vi "CFM_DAQ.vi"() -> ()   [LabVIEW 2012]
panel:
  in  "stop":bool
  out "reinicio":bool
  out "M54":bool
  out "M53":bool
  out "M52":bool
  out "M51":bool
  in  "ACTUADOR RECHAZO":bool
  out "M50":bool
  out "M49":bool
  out "M48":bool
  out "M47":bool
  out "M46":bool
  out "M45":bool
  out "M44":bool
  out "TAPA NOPESO":bool
  out "M43":bool
  out "M42":bool
  out "M41":bool
  out "M40":bool
  out "M39":bool
  out "M38":bool
  out "M37":bool
  out "M36":bool
  out "M35":bool
  out "M34":bool
  out "TARRO NOPESO":bool
  out "DEPOSITO NOPESO":bool
  out "TAPA NOCOLOR":bool
  out "TARRO NOCOLOR":bool
  out "DEPOSITO NOCOLOR":bool
  out "CILINDRO RECHAZO1":bool
  out "VASTAGO RECHAZO":bool
  out "PINZA CERRADA":bool
  in  "PINZA ABIERTA":bool
  out "CILINDRO RECHAZO":bool
  out "ESTRUCTURA RECHAZO":bool
  out "M33":bool
  out "M32":bool
  out "M31":bool
  out "M30":bool
  out "M29":bool
  out "M28":bool
  out "M27":bool
  out "M26":bool
  out "TAPA AZUL":bool
  out "M25":bool
  out "M24":bool
  out "TAPA TARRO ROJO":bool
  in  "CILINDRO MODULO6":bool
  in  "VASTAGO MODULO6":bool
  in  "MODULO6":bool
  out "M23":bool
  out "M22":bool
  out "M21":bool
  out "ANALIZANDO\nCC":bool
  out "M20":bool
  out "balanza2":bool
  out "M19":bool
  out "M18":bool
  out "M17":bool
  out "M16":bool
  out "M15":bool
  out "M14":bool
  out "M13":bool
  out "M12":bool
  out "M11":bool
  out "M10":bool
  out "M9":bool
  out "M8":bool
  out "M7":bool
  out "M6":bool
  out "M5":bool
  out "M4":bool
  out "M3":bool
  out "M2":bool
  out "M1":bool
  out "tapa neutrop":bool
  out "cilindro3 tapado":bool
  out "vastago3 tapado":bool
  out "vastago4 tapado":bool
  out "cilindro2 tapado":bool
  in  "vastago2 tapado":bool
  out "cilindro1 tapado":bool
  in  "vastago1 tapado":bool
  out "estructura tapado":bool
  out "tarro llenop":bool
  out "tarro vaciop1":bool
  out "cilindros tolva":bool
  out "perta tolva1":bool
  out "puerta tolva2":bool
  out "dep inferior":bool
  out "dep superior":bool
  out "tolva vacia":bool
  out "cuadroblanco":bool
  out "vastagoaux1":bool
  out "tarro vaciop":bool
  out "estructura1":bool
  out "CILINDRO NUEVO":bool
  out "TAPA NEUTRO":bool
  out "BALANZA1":bool
  in  "BASTAGO TAPAS":bool
  out "PUERTA TOLVA":bool
  out "CAJA LLENA":bool
  out "TARRO VACIO":bool
  in  "BPESO NO":bool
  in  "BPESO SI":bool
  in  "BNO COLOR":bool
  in  "BROJO":bool
  in  "BAZUL":bool
  in  "REINICIAR\nCONTEO":bool
  out "FINALIZADOS\nRECHAZADOS":dbl
  out "FINALIZADOS\nROJOS":dbl
  out "FINALIZADOS\nAZULES":dbl
  out "AZUL":bool
  out "ROJO":bool
  out "NO \nCOLOR":bool
  out "PESO\nNO":bool
  out "PESO\nSI":bool
  in  "RESET":bool
  in  "INICIO":bool
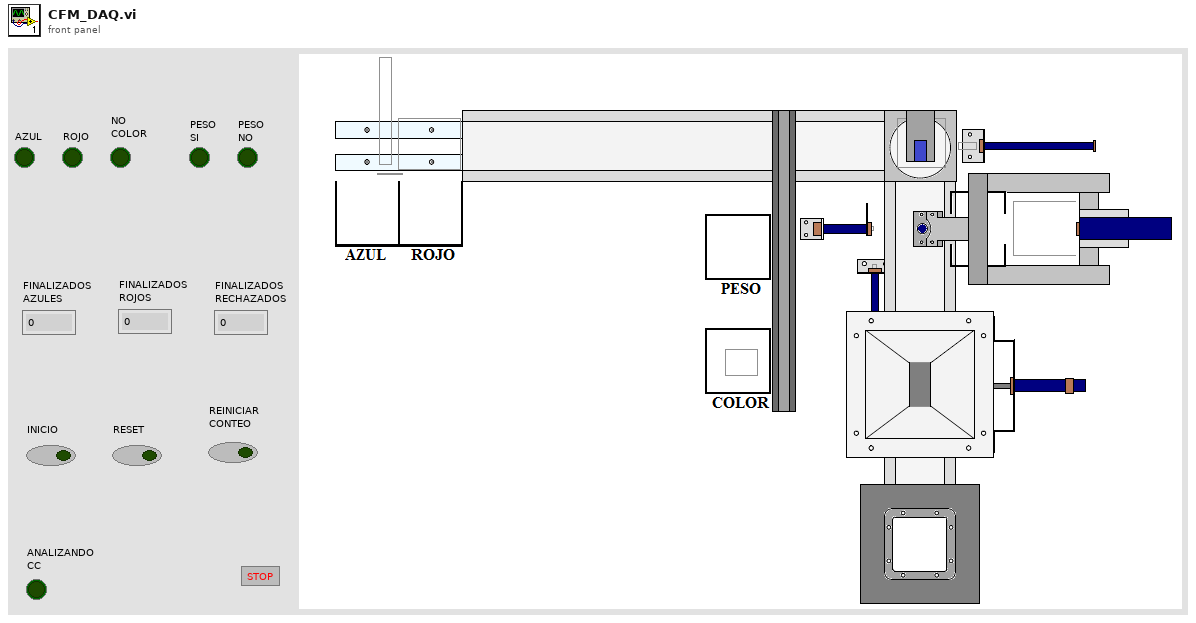
[diagram p1: front panel]
diagram:
  n1 = while {
    stop <- "stop" stop-if-true
    n2 = property on="M53" class="Bool (strict)"("Visible"=FALSE) -> ()  [unwired: 2 in, 2 out]
    n3 = property on="M54" class="Bool (strict)"("Visible"=FALSE) -> ()  [unwired: 2 in, 2 out]
    n4 = property on="M52" class="Bool (strict)"("Visible"=FALSE) -> ()  [unwired: 2 in, 2 out]
    n5 = property on="M48" class="Bool (strict)"("Visible"=FALSE) -> ()  [unwired: 2 in, 2 out]
    n6 = property on="M43" class="Bool (strict)"("Visible"=FALSE) -> ()  [unwired: 2 in, 2 out]
    n7 = property on="M47" class="Bool (strict)"("Visible"=FALSE) -> ()  [unwired: 2 in, 2 out]
    n8 = property on="M42" class="Bool (strict)"("Visible"=FALSE) -> ()  [unwired: 2 in, 2 out]
    n9 = property on="M41" class="Bool (strict)"("Visible"=FALSE) -> ()  [unwired: 2 in, 2 out]
    n10 = property on="M49" class="Bool (strict)"("Visible"=FALSE) -> ()  [unwired: 2 in, 2 out]
    n11 = property on="M40" class="Bool (strict)"("Visible"=FALSE) -> ()  [unwired: 2 in, 2 out]
    n12 = property on="M45" class="Bool (strict)"("Visible"=FALSE) -> ()  [unwired: 2 in, 2 out]
    n13 = property on="M46" class="Bool (strict)"("Visible"=FALSE) -> ()  [unwired: 2 in, 2 out]
    n14 = property on="reinicio" class="Bool (strict)"("Visible"=FALSE) -> ()  [unwired: 2 in, 2 out]
    n15 = property on="M24" class="Bool (strict)"("Visible"=FALSE) -> ()  [unwired: 2 in, 2 out]
    n16 = property on="M39" class="Bool (strict)"("Visible"=FALSE) -> ()  [unwired: 2 in, 2 out]
    n17 = property on="M44" class="Bool (strict)"("Visible"=FALSE) -> ()  [unwired: 2 in, 2 out]
    n18 = property on="M50" class="Bool (strict)"("Visible"=FALSE) -> ()  [unwired: 2 in, 2 out]
    n19 = property on="M25" class="Bool (strict)"("Visible"=FALSE) -> ()  [unwired: 2 in, 2 out]
    n20 = property on="M37" class="Bool (strict)"("Visible"=FALSE) -> ()  [unwired: 2 in, 2 out]
    n21 = property on="M38" class="Bool (strict)"("Visible"=FALSE) -> ()  [unwired: 2 in, 2 out]
    n22 = property on="M23" class="Bool (strict)"("Visible"=FALSE) -> ()  [unwired: 2 in, 2 out]
    n23 = property on="M22" class="Bool (strict)"("Visible"=FALSE) -> ()  [unwired: 2 in, 2 out]
    n24 = property on="M51" class="Bool (strict)"("Visible"=FALSE) -> ()  [unwired: 2 in, 2 out]
    n25 = property on="M36" class="Bool (strict)"("Visible"=FALSE) -> ()  [unwired: 2 in, 2 out]
    n26 = property on="M21" class="Bool (strict)"("Visible"=FALSE) -> ()  [unwired: 2 in, 2 out]
    n27 = property on="M27" class="Bool (strict)"("Visible"=FALSE) -> ()  [unwired: 2 in, 2 out]
    n28 = property on="M33" class="Bool (strict)"("Visible"=FALSE) -> ()  [unwired: 2 in, 2 out]
    n29 = property on="M2" class="Bool (strict)"("Visible"=FALSE) -> ()  [unwired: 2 in, 2 out]
    n30 = property on="M26" class="Bool (strict)"("Visible"=FALSE) -> ()  [unwired: 2 in, 2 out]
    n31 = property on="M35" class="Bool (strict)"("Visible"=FALSE) -> ()  [unwired: 2 in, 2 out]
    n32 = property on="M1" class="Bool (strict)"("Visible"=FALSE) -> ()  [unwired: 2 in, 2 out]
    n33 = property on="M32" class="Bool (strict)"("Visible"=FALSE) -> ()  [unwired: 2 in, 2 out]
    n34 = property on="M34" class="Bool (strict)"("Visible"=FALSE) -> ()  [unwired: 2 in, 2 out]
    n35 = property on="M13" class="Bool (strict)"("Visible"=FALSE) -> ()  [unwired: 2 in, 2 out]
    n36 = property on="M20" class="Bool (strict)"("Visible"=FALSE) -> ()  [unwired: 2 in, 2 out]
    n37 = property on="M29" class="Bool (strict)"("Visible"=FALSE) -> ()  [unwired: 2 in, 2 out]
    n38 = property on="M15" class="Bool (strict)"("Visible"=FALSE) -> ()  [unwired: 2 in, 2 out]
    n39 = property on="M28" class="Bool (strict)"("Visible"=FALSE) -> ()  [unwired: 2 in, 2 out]
    n40 = property on="M5" class="Bool (strict)"("Visible"=FALSE) -> ()  [unwired: 2 in, 2 out]
    n41 = property on="M3" class="Bool (strict)"("Visible"=FALSE) -> ()  [unwired: 2 in, 2 out]
    n42 = property on="M18" class="Bool (strict)"("Visible"=FALSE) -> ()  [unwired: 2 in, 2 out]
    n43 = property on="M19" class="Bool (strict)"("Visible"=FALSE) -> ()  [unwired: 2 in, 2 out]
    n44 = property on="M8" class="Bool (strict)"("Visible"=FALSE) -> ()  [unwired: 2 in, 2 out]
    n45 = property on="M7" class="Bool (strict)"("Visible"=FALSE) -> ()  [unwired: 2 in, 2 out]
    n46 = property on="M30" class="Bool (strict)"("Visible"=FALSE) -> ()  [unwired: 2 in, 2 out]
    n47 = property on="M6" class="Bool (strict)"("Visible"=FALSE) -> ()  [unwired: 2 in, 2 out]
    n48 = property on="M9" class="Bool (strict)"("Visible"=FALSE) -> ()  [unwired: 2 in, 2 out]
    n49 = property on="M17" class="Bool (strict)"("Visible"=FALSE) -> ()  [unwired: 2 in, 2 out]
    n50 = property on="M4" class="Bool (strict)"("Visible"=FALSE) -> ()  [unwired: 2 in, 2 out]
    n51 = property on="M10" class="Bool (strict)"("Visible"=FALSE) -> ()  [unwired: 2 in, 2 out]
    n52 = property on="M11" class="Bool (strict)"("Visible"=FALSE) -> ()  [unwired: 2 in, 2 out]
    n53 = property on="M14" class="Bool (strict)"("Visible"=FALSE) -> ()  [unwired: 2 in, 2 out]
    n54 = property on="M16" class="Bool (strict)"("Visible"=FALSE) -> ()  [unwired: 2 in, 2 out]
    n55 = property on="M12" class="Bool (strict)"("Visible"=FALSE) -> ()  [unwired: 2 in, 2 out]
    n56 = property on="M31" class="Bool (strict)"("Visible"=FALSE) -> ()  [unwired: 2 in, 2 out]
    n57 = property on="ACTUADOR RECHAZO" class="Bool (strict)"() -> ("Top"=w101:i32)  [unwired: 2 in, 2 out]
    n58 = property on="ACTUADOR RECHAZO" class="Bool (strict)"() -> ("Top"=w86:i32)  [unwired: 2 in, 2 out]
    n59 = local read "BNO COLOR"() -> (w140:bool)
    n60 = property on="ACTUADOR RECHAZO" class="Bool (strict)"() -> ("Top"=w116:i32)  [unwired: 2 in, 2 out]
    n61 = property on="ACTUADOR RECHAZO" class="Bool (strict)"() -> ("Top"=w173:i32)  [unwired: 2 in, 2 out]
    n62 = property on="ACTUADOR RECHAZO" class="Bool (strict)"() -> ("Top"=w158:i32)  [unwired: 2 in, 2 out]
    n63 = property on="VASTAGO MODULO6" class="Bool (strict)"() -> ("Top"=w251:i32)  [unwired: 2 in, 2 out]
    n64 = property on="VASTAGO MODULO6" class="Bool (strict)"() -> ("Top"=w214:i32)  [unwired: 2 in, 2 out]
    n65 = property on="VASTAGO MODULO6" class="Bool (strict)"() -> ("Top"=w209:i32)  [unwired: 2 in, 2 out]
    n66 = property on="VASTAGO MODULO6" class="Bool (strict)"() -> ("Top"=w256:i32)  [unwired: 2 in, 2 out]
    n67 = local read "BPESO NO"() -> (w141:bool)
    n68 = local read "BPESO NO"() -> (w187:bool)
    n69 = property on="TAPA TARRO ROJO" class="Bool (strict)"() -> ("Left"=w261:i32)  [unwired: 2 in, 2 out]
    n70 = property on="PINZA CERRADA" class="Bool (strict)"() -> ("Top"=w96:i32)  [unwired: 2 in, 2 out]
    n71 = property on="PINZA CERRADA" class="Bool (strict)"() -> ("Top"=w148:i32)  [unwired: 2 in, 2 out]
    n72 = property on="PINZA CERRADA" class="Bool (strict)"() -> ("Top"=w106:i32)  [unwired: 2 in, 2 out]
    n73 = property on="PINZA CERRADA" class="Bool (strict)"() -> ("Top"=w91:i32)  [unwired: 2 in, 2 out]
    n74 = property on="vastago4 tapado" class="Bool (strict)"() -> ("Top"=w319:i32)  [unwired: 2 in, 2 out]
    n75 = property on="PINZA CERRADA" class="Bool (strict)"() -> ("Top"=w168:i32)  [unwired: 2 in, 2 out]
    n76 = property on="PINZA CERRADA" class="Bool (strict)"() -> ("Top"=w163:i32)  [unwired: 2 in, 2 out]
    n77 = property on="vastago4 tapado" class="Bool (strict)"() -> ("Top"=w314:i32)  [unwired: 2 in, 2 out]
    n78 = property on="TAPA NOCOLOR" class="Bool (strict)"() -> ("Left"=w178:i32)  [unwired: 2 in, 2 out]
    n79 = property on="PINZA CERRADA" class="Bool (strict)"() -> ("Top"=w111:i32)  [unwired: 2 in, 2 out]
    n80 = property on="BASTAGO TAPAS" class="Bool (strict)"() -> ("Left"=w324:i32)  [unwired: 2 in, 2 out]
    n81 = local read "BNO COLOR"() -> (w188:bool)
    n82 = property on="CILINDRO NUEVO" class="Bool (strict)"() -> ("Left"=w309:i32)  [unwired: 2 in, 2 out]
    n83 = property on="vastago3 tapado" class="Bool (strict)"() -> ("Top"=w299:i32)  [unwired: 2 in, 2 out]
    n84 = property on="PINZA CERRADA" class="Bool (strict)"() -> ("Top"=w153:i32)  [unwired: 2 in, 2 out]
    n85 = property on="TAPA NOPESO" class="Bool (strict)"() -> ("Left"=w121:i32)  [unwired: 2 in, 2 out]
    n86 = property on="TAPA NEUTRO" class="Bool (strict)"() -> ("Top"=w294:i32)  [unwired: 2 in, 2 out]
    n87 = property on="balanza2" class="Bool (strict)"() -> ("Left"=w128:i32)  [unwired: 2 in, 2 out]
    n88 = property on="TAPA NEUTRO" class="Bool (strict)"() -> ("Top"=w284:i32)  [unwired: 2 in, 2 out]
    n89 = property on="tapa neutrop" class="Bool (strict)"() -> ("Top"=w304:i32)  [unwired: 2 in, 2 out]
    n90 = property on="PUERTA TOLVA" class="Bool (strict)"() -> ("Left"=w349:i32)  [unwired: 2 in, 2 out]
    n91 = property on="PUERTA TOLVA" class="Bool (strict)"() -> ("Left"=w344:i32)  [unwired: 2 in, 2 out]
    n92 = call "DAQ Assistant"() -> ("data"=w76:bool[])  [unwired: 17 in, 2 out]
    n93 = property on="TARRO VACIO" class="Bool (strict)"() -> ("Top"=w354:i32)  [unwired: 2 in, 2 out]
    n94 = property on="vastagoaux1" class="Bool (strict)"() -> ("Top"=w364:i32)  [unwired: 2 in, 2 out]
    n95 = local read "BPESO SI"() -> (w243:bool)
    n96 = local read "BPESO NO"() -> (w143:bool)
    n97 = property on="balanza2" class="Bool (strict)"() -> ("Left"=w138:i32)  [unwired: 2 in, 2 out]
    n98 = local read "BPESO SI"() -> (w249:bool)
    n99 = property on="vastagoaux1" class="Bool (strict)"() -> ("Top"=w369:i32)  [unwired: 2 in, 2 out]
    n100 = property on="vastagoaux1" class="Bool (strict)"() -> ("Top"=w359:i32)  [unwired: 2 in, 2 out]
    n101 = property on="puerta tolva2" class="Bool (strict)"() -> ("Left"=w339:i32)  [unwired: 2 in, 2 out]
    n102 = property on="puerta tolva2" class="Bool (strict)"() -> ("Left"=w334:i32)  [unwired: 2 in, 2 out]
    n103 = property on="TAPA AZUL" class="Bool (strict)"() -> ("Left"=w224:i32)  [unwired: 2 in, 2 out]
    n104 = property on="CAJA LLENA" class="Bool (strict)"() -> ("Top"=w329:i32)  [unwired: 2 in, 2 out]
    n105 = property on="BALANZA1" class="Bool (strict)"() -> ("Top"=w289:i32)  [unwired: 2 in, 2 out]
    n106 = property on="MODULO6" class="Bool (strict)"() -> ("Left"=w219:i32)  [unwired: 2 in, 2 out]
    n107 = property on="MODULO6" class="Bool (strict)"() -> ("Left"=w204:i32)  [unwired: 2 in, 2 out]
    n108 = local read "BAZUL"() -> (w244:bool)
    n109 = property on="balanza2" class="Bool (strict)"() -> ("Left"=w133:i32)  [unwired: 2 in, 2 out]
    n110 = local read "BROJO"() -> (w248:bool)
    n111 = property on="balanza2" class="Bool (strict)"() -> ("Left"=w239:i32)  [unwired: 2 in, 2 out]
    n112 = property on="balanza2" class="Bool (strict)"() -> ("Left"=w278:i32)  [unwired: 2 in, 2 out]
    n113 = property on="balanza2" class="Bool (strict)"() -> ("Left"=w183:i32)  [unwired: 2 in, 2 out]
    n114 = property on="balanza2" class="Bool (strict)"() -> ("Left"=w229:i32)  [unwired: 2 in, 2 out]
    n115 = property on="balanza2" class="Bool (strict)"() -> ("Left"=w195:i32)  [unwired: 2 in, 2 out]
    n116 = property on="balanza2" class="Bool (strict)"() -> ("Left"=w266:i32)  [unwired: 2 in, 2 out]
    n117 = property on="balanza2" class="Bool (strict)"() -> ("Left"=w234:i32)  [unwired: 2 in, 2 out]
    n118 = property on="balanza2" class="Bool (strict)"() -> ("Left"=w190:i32)  [unwired: 2 in, 2 out]
    n119 = property on="balanza2" class="Bool (strict)"() -> ("Left"=w271:i32)  [unwired: 2 in, 2 out]
    n120 = local read "reinicio"() -> (w82:bool)
    n121 = local read "INICIO"() -> (w83:bool)
    n122 = Not(x=w187) -> (.not. x?=w199:bool)
    n123 = local read "M46"() -> (w125:bool)
    n124 = And(x=w141, y=w140) -> (x .and. y?=w142:bool)
    n125 = Less?(x=w138, y=965) -> (x < y?=w139:bool)
    n126 = local read "M52"() -> (w98:bool)
    n127 = local read "M47"() -> (w123:bool)
    n128 = local read "M45"() -> (w130:bool)
    n129 = local read "M43"() -> (w150:bool)
    n130 = local read "M50"() -> (w108:bool)
    n131 = local read "M44"() -> (w135:bool)
    n132 = local read "M51"() -> (w103:bool)
    n133 = local read "M54"() -> (w88:bool)
    n134 = local read "M19"() -> (w281:bool)
    n135 = local read "M25"() -> (w253:bool)
    n136 = local read "M26"() -> (w241:bool)
    n137 = local read "M36"() -> (w185:bool)
    n138 = local read "M37"() -> (w180:bool)
    n139 = Greater?(x=w128, y=977) -> (0:w129:bool)
    n140 = local read "M53"() -> (w93:bool)
    n141 = local read "M28"() -> (w231:bool)
    n142 = local read "M48"() -> (w118:bool)
    n143 = local read "M10"() -> (w326:bool)
    n144 = local read "M14"() -> (w306:bool)
    n145 = local read "M16"() -> (w296:bool)
    n146 = local read "M20"() -> (w276:bool)
    n147 = local read "M30"() -> (w221:bool)
    n148 = local read "M31"() -> (w216:bool)
    n149 = local read "M33"() -> (w206:bool)
    n150 = local read "M39"() -> (w170:bool)
    n151 = local read "M40"() -> (w165:bool)
    n152 = local read "M23"() -> (w263:bool)
    n153 = local read "M29"() -> (w226:bool)
    n154 = local read "M34"() -> (w197:bool)
    n155 = local read "M41"() -> (w160:bool)
    n156 = local read "M12"() -> (w316:bool)
    n157 = local read "M19"() -> (w246:bool)
    n158 = local read "M32"() -> (w211:bool)
    n159 = local read "M19"() -> (w201:bool)
    n160 = local read "M38"() -> (w175:bool)
    n161 = local read "M49"() -> (w113:bool)
    n162 = local read "M11"() -> (w321:bool)
    n163 = local read "M17"() -> (w291:bool)
    n164 = local read "M18"() -> (w286:bool)
    n165 = local read "M22"() -> (w268:bool)
    n166 = local read "M24"() -> (w258:bool)
    n167 = local read "M27"() -> (w236:bool)
    n168 = local read "M35"() -> (w192:bool)
    n169 = local read "M42"() -> (w155:bool)
    n170 = local read "M19"() -> (w145:bool)
    n171 = local read "M2"() -> (w366:bool)
    n172 = local read "M15"() -> (w301:bool)
    n173 = local read "M1"() -> (w371:bool)
    n174 = local read "M21"() -> (w273:bool)
    n175 = local read "M4"() -> (w356:bool)
    n176 = local read "M13"() -> (w311:bool)
    n177 = local read "M6"() -> (w346:bool)
    n178 = local read "M8"() -> (w336:bool)
    n179 = local read "M3"() -> (w361:bool)
    n180 = local read "M5"() -> (w351:bool)
    n181 = local read "M9"() -> (w331:bool)
    n182 = Less?(x=w133, y=900) -> (x < y?=w134:bool)
    n183 = local read "M7"() -> (w341:bool)
    n184 = Equal?(x=420, y=w369) -> (x = y?=w370:bool)
    n185 = Less?(x=w121, y=737) -> (x < y?=w122:bool)
    n186 = property on="BAZUL" class="Bool (strict)"("Visible"=FALSE) -> ()  [unwired: 2 in, 2 out]
    n187 = Greater?(x=w214, y=55) -> (0:w215:bool)
    n188 = Less?(x=w148, y=317) -> (x < y?=w149:bool)
    n189 = Greater?(x=w96, y=396) -> (0:w97:bool)
    n190 = property on="BROJO" class="Bool (strict)"("Visible"=FALSE) -> ()  [unwired: 2 in, 2 out]
    n191 = And(x=w248, y=w249) -> (x .and. y?=w280:bool)
    n192 = Less?(x=w294, y=67) -> (x < y?=w295:bool)
    n193 = And(x=w244, y=w243) -> (x .and. y?=w245:bool)
    n194 = Less?(x=w224, y=426) -> (x < y?=w225:bool)
    n195 = Greater?(x=w158, y=219) -> (0:w159:bool)
    n196 = Less?(x=w116, y=6) -> (x < y?=w117:bool)
    n197 = Less?(x=w106, y=317) -> (x < y?=w107:bool)
    n198 = Less?(x=w251, y=-10) -> (x < y?=w252:bool)
    n199 = Less?(x=w178, y=737) -> (x < y?=w179:bool)
    n200 = Greater?(x=w86, y=219) -> (0:w87:bool)
    n201 = Less?(x=w324, y=911) -> (x < y?=w325:bool)
    n202 = Greater?(x=w304, y=367) -> (0:w305:bool)
    n203 = Less?(x=w234, y=900) -> (x < y?=w235:bool)
    n204 = Greater?(x=w229, y=977) -> (0:w230:bool)
    n205 = Greater?(x=w204, y=377) -> (0:w205:bool)
    n206 = Less?(x=w163, y=317) -> (x < y?=w164:bool)
    n207 = Greater?(x=w111, y=396) -> (0:w112:bool)
    n208 = Greater?(x=w359, y=383) -> (0:w360:bool)
    n209 = Less?(x=w354, y=252) -> (x < y?=w355:bool)
    n210 = Greater?(x=w319, y=258) -> (0:w320:bool)
    n211 = Less?(x=w278, y=965) -> (x < y?=w275:bool)
    n212 = Greater?(x=w256, y=38) -> (0:w257:bool)
    n213 = And(x=w188, y=w199) -> (x .and. y?=w200:bool)
    n214 = Less?(x=w91, y=317) -> (x < y?=w92:bool)
    n215 = Less?(x=w261, y=426) -> (x < y?=w262:bool)
    n216 = Less?(x=w239, y=965) -> (x < y?=w240:bool)
    n217 = Less?(x=w219, y=316) -> (x < y?=w220:bool)
    n218 = Less?(x=w209, y=10) -> (x < y?=w210:bool)
    n219 = Less?(x=w195, y=965) -> (x < y?=w196:bool)
    n220 = Less?(x=w190, y=900) -> (x < y?=w191:bool)
    n221 = Greater?(x=w183, y=977) -> (0:w184:bool)
    n222 = Less?(x=w173, y=6) -> (x < y?=w174:bool)
    n223 = Greater?(x=w153, y=396) -> (0:w154:bool)
    n224 = Or(x=w143, y=w142) -> (x .or. y?=w144:bool)
    n225 = Less?(x=w344, y=931) -> (x < y?=w345:bool)
    n226 = Less?(x=w314, y=227) -> (x < y?=w315:bool)
    n227 = Less?(x=w289, y=109) -> (x < y?=w290:bool)
    n228 = Greater?(x=w266, y=977) -> (0:w267:bool)
    n229 = Greater?(x=w168, y=396) -> (0:w169:bool)
    n230 = Greater?(x=w101, y=100) -> (0:w102:bool)
    n231 = Less?(x=w364, y=386) -> (x < y?=w365:bool)
    n232 = Less?(x=w339, y=425) -> (x < y?=w340:bool)
    n233 = Less?(x=w329, y=97) -> (x < y?=w330:bool)
    n234 = Less?(x=w284, y=16) -> (x < y?=w285:bool)
    n235 = Greater?(x=w334, y=449) -> (0:w335:bool)
    n236 = Less?(x=w309, y=870) -> (x < y?=w310:bool)
    n237 = Greater?(x=w349, y=950) -> (0:w350:bool)
    n238 = Less?(x=w299, y=207) -> (x < y?=w300:bool)
    n239 = Less?(x=w271, y=900) -> (x < y?=w272:bool)
    n240 = local read "RESET"() -> (w62:bool)
    n241 = Or(x=w83, y=w82) -> (x .or. y?=w84:bool)
    n242 = And(x=w296, y=w295) -> (x .and. y?=w297:bool)
    n243 = And(x=w180, y=w179) -> (x .and. y?=w181:bool)
    n244 = And(x=w371, y=w370) -> (x .and. y?=w372:bool)
    n245 = And(x=w306, y=w305) -> (x .and. y?=w307:bool)
    n246 = And(x=w253, y=w252) -> (x .and. y?=w254:bool)
    n247 = And(x=w165, y=w164) -> (x .and. y?=w166:bool)
    n248 = And(x=w150, y=w149) -> (x .and. y?=w151:bool)
    n249 = And(x=w130, y=w134) -> (x .and. y?=w131:bool)
    n250 = And(x=w125, y=w129) -> (x .and. y?=w126:bool)
    n251 = And(x=w98, y=w97) -> (x .and. y?=w99:bool)
    n252 = And(x=w356, y=w355) -> (x .and. y?=w357:bool)
    n253 = And(x=w246, y=w245) -> (x .and. y?=w247:bool)
    n254 = And(x=w241, y=w240) -> (x .and. y?=w242:bool)
    n255 = And(x=w197, y=w196) -> (x .and. y?=w198:bool)
    n256 = And(x=w185, y=w184) -> (x .and. y?=w186:bool)
    n257 = And(x=w135, y=w139) -> (x .and. y?=w136:bool)
    n258 = And(x=w366, y=w365) -> (x .and. y?=w367:bool)
    n259 = And(x=w346, y=w345) -> (x .and. y?=w347:bool)
    n260 = And(x=w291, y=w290) -> (x .and. y?=w292:bool)
    n261 = And(x=w263, y=w262) -> (x .and. y?=w264:bool)
    n262 = And(x=w211, y=w210) -> (x .and. y?=w212:bool)
    n263 = And(x=w170, y=w169) -> (x .and. y?=w171:bool)
    n264 = And(x=w123, y=w122) -> (x .and. y?=w124:bool)
    n265 = And(x=w326, y=w325) -> (x .and. y?=w327:bool)
    n266 = And(x=w321, y=w320) -> (x .and. y?=w322:bool)
    n267 = And(x=w316, y=w315) -> (x .and. y?=w317:bool)
    n268 = And(x=w286, y=w285) -> (x .and. y?=w287:bool)
    n269 = And(x=w281, y=w280) -> (x .and. y?=w282:bool)
    n270 = And(x=w276, y=w275) -> (x .and. y?=w279:bool)
    n271 = And(x=w268, y=w267) -> (x .and. y?=w269:bool)
    n272 = And(x=w258, y=w257) -> (x .and. y?=w259:bool)
    n273 = And(x=w231, y=w230) -> (x .and. y?=w232:bool)
    n274 = And(x=w226, y=w225) -> (x .and. y?=w227:bool)
    n275 = And(x=w221, y=w220) -> (x .and. y?=w222:bool)
    n276 = And(x=w201, y=w200) -> (x .and. y?=w202:bool)
    n277 = And(x=w192, y=w191) -> (x .and. y?=w193:bool)
    n278 = And(x=w160, y=w159) -> (x .and. y?=w161:bool)
    n279 = And(x=w118, y=w117) -> (x .and. y?=w119:bool)
    n280 = And(x=w108, y=w107) -> (x .and. y?=w109:bool)
    n281 = And(x=w93, y=w92) -> (x .and. y?=w94:bool)
    n282 = And(x=w88, y=w87) -> (x .and. y?=w89:bool)
    n283 = And(x=w361, y=w360) -> (x .and. y?=w362:bool)
    n284 = And(x=w351, y=w350) -> (x .and. y?=w352:bool)
    n285 = And(x=w336, y=w335) -> (x .and. y?=w337:bool)
    n286 = And(x=w331, y=w330) -> (x .and. y?=w332:bool)
    n287 = And(x=w236, y=w235) -> (x .and. y?=w237:bool)
    n288 = And(x=w216, y=w215) -> (x .and. y?=w217:bool)
    n289 = And(x=w206, y=w205) -> (x .and. y?=w207:bool)
    n290 = And(x=w175, y=w174) -> (x .and. y?=w176:bool)
    n291 = And(x=w155, y=w154) -> (x .and. y?=w156:bool)
    n292 = And(x=w341, y=w340) -> (x .and. y?=w342:bool)
    n293 = And(x=w311, y=w310) -> (x .and. y?=w312:bool)
    n294 = And(x=w273, y=w272) -> (x .and. y?=w274:bool)
    n295 = And(x=w103, y=w102) -> (x .and. y?=w104:bool)
    n296 = And(x=w301, y=w300) -> (x .and. y?=w302:bool)
    n297 = And(x=w113, y=w112) -> (x .and. y?=w114:bool)
    n298 = And(x=w145, y=w144) -> (x .and. y?=w146:bool)
    n299 = Index Array(array=w76, index=0) -> (element=w77:bool)
    n300 = Index Array(array=w76, index=1 ("index 2")) -> (element=w81:bool)
    n301 = Index Array(array=w76, index=2) -> (element=w80:bool)
    n302 = Index Array(array=w76, index=3) -> (element=w79:bool)
    n303 = Index Array(array=w76, index=4) -> (element=w78:bool)
    n304 = case shown="True" w217 {
      frame False {
      }
      frame True {
        n305 = local read "FINALIZADOS\nAZULES"() -> (w873:dbl)
        n306 = Increment(x=w873) -> (x+1=w872:dbl)
        n307 = local write "FINALIZADOS\nAZULES"(w872) -> ()
        n308 = while {
          stop <- w874 stop-if-true
          n309 = property on="VASTAGO MODULO6" class="Bool (strict)"() -> ("Top"=w882:i32)  [unwired: 2 in, 2 out]
          n310 = Subtract(x=w882, y=2) -> (x-y=w880:i32)
          n311 = property on="VASTAGO MODULO6" class="Bool (strict)"("Top"=w880) -> ()  [unwired: 2 in, 2 out]
          n312 = Wait (ms)(milliseconds to wait=u32 0) -> ()  [unwired: 1 out]
          n313 = local read "RESET"() -> (w875:bool)
          n314 = property on="VASTAGO MODULO6" class="Bool (strict)"() -> ("Top"=w878:i32)  [unwired: 2 in, 2 out]
          n315 = Less?(x=w878, y=-10) -> (x < y?=w876:bool)
          n316 = Or(x=w876, y=w875) -> (x .or. y?=w874:bool)
        }
        n317 = local write "AZUL"(FALSE ("AZUL")) -> ()
        n318 = local write "PESO\nSI"(FALSE ("PESO\nSI")) -> ()
        n319 = local write "M31"(FALSE ("M31")) -> ()
        n320 = local write "M32"(TRUE ("M32")) -> ()
      }
    }
    n321 = case shown="True" w84 {
      frame False {
      }
      frame True {
        n322 = property on="TARRO VACIO" class="Bool (strict)"("Visible"=TRUE) -> ()  [unwired: 2 in, 2 out]
        n323 = property on="TAPA NEUTRO" class="Bool (strict)"("Visible"=TRUE) -> ()  [unwired: 2 in, 2 out]
        n324 = property on="estructura1" class="Bool (strict)"("Visible"=TRUE) -> ()  [unwired: 2 in, 2 out]
        n325 = property on="tarro vaciop" class="Bool (strict)"("Visible"=TRUE) -> ()  [unwired: 2 in, 2 out]
        n326 = property on="vastagoaux1" class="Bool (strict)"("Visible"=TRUE) -> ()  [unwired: 2 in, 2 out]
        n327 = property on="cuadroblanco" class="Bool (strict)"("Visible"=TRUE) -> ()  [unwired: 2 in, 2 out]
        n328 = property on="vastagoaux1" class="Bool (strict)"("Top"=420 ("Position:Top")) -> ()  [unwired: 2 in, 2 out]
        n329 = property on="TAPA NEUTRO" class="Bool (strict)"("Top"=96 ("Position:Top")) -> ()  [unwired: 2 in, 2 out]
        n330 = property on="TARRO VACIO" class="Bool (strict)"("Top"=412 ("Position:Top")) -> ()  [unwired: 2 in, 2 out]
        n331 = property on="CAJA LLENA" class="Bool (strict)"("Top"=250 ("Position:Top")) -> ()  [unwired: 2 in, 2 out]
        n332 = property on="PUERTA TOLVA" class="Bool (strict)"("Left"=929 ("Position:Left")) -> ()  [unwired: 2 in, 2 out]
        n333 = property on="BALANZA1" class="Bool (strict)"("Top"=146 ("Position:Top")) -> ()  [unwired: 2 in, 2 out]
        n334 = property on="CAJA LLENA" class="Bool (strict)"("Visible"=FALSE) -> ()  [unwired: 2 in, 2 out]
        n335 = property on="dep inferior" class="Bool (strict)"("Visible"=FALSE) -> ()  [unwired: 2 in, 2 out]
        n336 = property on="dep superior" class="Bool (strict)"("Visible"=FALSE) -> ()  [unwired: 2 in, 2 out]
        n337 = property on="cilindros tolva" class="Bool (strict)"("Visible"=FALSE) -> ()  [unwired: 2 in, 2 out]
        n338 = property on="puerta tolva2" class="Bool (strict)"("Visible"=FALSE) -> ()  [unwired: 2 in, 2 out]
        n339 = property on="perta tolva1" class="Bool (strict)"("Visible"=FALSE) -> ()  [unwired: 2 in, 2 out]
        n340 = local write "M1"(TRUE ("M1")) -> ()
        n341 = property on="CILINDRO NUEVO" class="Bool (strict)"("Left"=869 ("Position:Left")) -> ()  [unwired: 2 in, 2 out]
        n342 = property on="BASTAGO TAPAS" class="Bool (strict)"("Left"=973 ("Position:Left")) -> ()  [unwired: 2 in, 2 out]
        n343 = property on="tarro vaciop" class="Bool (strict)"("Top"=358 ("Position:Top")) -> ()  [unwired: 2 in, 2 out]
        n344 = property on="TAPA NEUTRO" class="Bool (strict)"("Left"=980 ("Position:Left")) -> ()  [unwired: 2 in, 2 out]
        n345 = property on="puerta tolva2" class="Bool (strict)"("Left"=450 ("Position:Left")) -> ()  [unwired: 2 in, 2 out]
        n346 = property on="perta tolva1" class="Bool (strict)"("Left"=450 ("Position:Left")) -> ()  [unwired: 2 in, 2 out]
        n347 = local write "reinicio"(FALSE ("reinicio")) -> ()
        n348 = property on="tolva vacia" class="Bool (strict)"("Visible"=FALSE) -> ()  [unwired: 2 in, 2 out]
        n349 = property on="tarro vaciop1" class="Bool (strict)"("Visible"=FALSE) -> ()  [unwired: 2 in, 2 out]
        n350 = property on="tarro llenop" class="Bool (strict)"("Visible"=FALSE) -> ()  [unwired: 2 in, 2 out]
        n351 = property on="estructura tapado" class="Bool (strict)"("Visible"=FALSE) -> ()  [unwired: 2 in, 2 out]
        n352 = property on="tapa neutrop" class="Bool (strict)"("Visible"=FALSE) -> ()  [unwired: 2 in, 2 out]
        n353 = property on="vastago1 tapado" class="Bool (strict)"("Visible"=FALSE) -> ()  [unwired: 2 in, 2 out]
        n354 = property on="tapa neutrop" class="Bool (strict)"("Top"=345 ("Position:Top")) -> ()  [unwired: 2 in, 2 out]
        n355 = property on="tapa neutrop" class="Bool (strict)"("Left"=527 ("Position:Left")) -> ()  [unwired: 2 in, 2 out]
        n356 = property on="vastago1 tapado" class="Bool (strict)"("Left"=361 ("Position:Left")) -> ()  [unwired: 2 in, 2 out]
        n357 = property on="vastago3 tapado" class="Bool (strict)"("Top"=206 ("Position:Top")) -> ()  [unwired: 2 in, 2 out]
        n358 = property on="vastago2 tapado" class="Bool (strict)"("Left"=626 ("Position:Left")) -> ()  [unwired: 2 in, 2 out]
        n359 = property on="vastago4 tapado" class="Bool (strict)"("Top"=226 ("Position:Top")) -> ()  [unwired: 2 in, 2 out]
        n360 = property on="cilindro1 tapado" class="Bool (strict)"("Visible"=FALSE) -> ()  [unwired: 2 in, 2 out]
        n361 = property on="vastago2 tapado" class="Bool (strict)"("Visible"=FALSE) -> ()  [unwired: 2 in, 2 out]
        n362 = property on="cilindro2 tapado" class="Bool (strict)"("Visible"=FALSE) -> ()  [unwired: 2 in, 2 out]
        n363 = property on="vastago3 tapado" class="Bool (strict)"("Visible"=FALSE) -> ()  [unwired: 2 in, 2 out]
        n364 = property on="cilindro3 tapado" class="Bool (strict)"("Visible"=FALSE) -> ()  [unwired: 2 in, 2 out]
        n365 = property on="vastago4 tapado" class="Bool (strict)"("Visible"=FALSE) -> ()  [unwired: 2 in, 2 out]
        n366 = property on="balanza2" class="Bool (strict)"("Left"=978 ("Position:Left")) -> ()  [unwired: 2 in, 2 out]
      }
    }
    n367 = case shown="True" w372 {
      frame False {
      }
      frame True {
        n368 = while {
          stop <- w1356 stop-if-true
          n369 = property on="vastagoaux1" class="Bool (strict)"() -> ("Top"=w1362:i32)  [unwired: 2 in, 2 out]
          n370 = Subtract(x=w1362, y=1) -> (x-y=w1363:i32)
          n371 = property on="vastagoaux1" class="Bool (strict)"("Top"=w1363) -> ()  [unwired: 2 in, 2 out]
          n372 = Wait (ms)(milliseconds to wait=u32 0) -> ()  [unwired: 1 out]
          n373 = property on="vastagoaux1" class="Bool (strict)"() -> ("Top"=w1360:i32)  [unwired: 2 in, 2 out]
          n374 = local read "RESET"() -> (w1357:bool)
          n375 = Less?(x=w1360, y=386) -> (x < y?=w1358:bool)
          n376 = Or(x=w1358, y=w1357) -> (x .or. y?=w1356:bool)
        }
        n377 = local write "M1"(FALSE ("M1")) -> ()
        n378 = local write "M2"(TRUE ("M2")) -> ()
      }
    }
    n379 = case shown="True" w367 {
      frame False {
      }
      frame True {
        n380 = while {
          stop <- w1341 stop-if-true
          n381 = property on="vastagoaux1" class="Bool (strict)"() -> ("Top"=w1352:i32)  [unwired: 2 in, 2 out]
          n382 = Add(x=w1352, y=1) -> (x+y=w1350:i32)
          n383 = property on="vastagoaux1" class="Bool (strict)"("Top"=w1350) -> ()  [unwired: 2 in, 2 out]
          n384 = property on="tarro vaciop" class="Bool (strict)"() -> ("Top"=w1349:i32)  [unwired: 2 in, 2 out]
          n385 = Add(x=w1349, y=1) -> (x+y=w1347:i32)
          n386 = property on="tarro vaciop" class="Bool (strict)"("Top"=w1347) -> ()  [unwired: 2 in, 2 out]
          n387 = Wait (ms)(milliseconds to wait=u32 0) -> ()  [unwired: 1 out]
          n388 = property on="vastagoaux1" class="Bool (strict)"() -> ("Top"=w1346:i32)  [unwired: 2 in, 2 out]
          n389 = local read "RESET"() -> (w1342:bool)
          n390 = Greater?(x=w1346, y=419) -> (0:w1343:bool)
          n391 = Or(x=w1343, y=w1342) -> (x .or. y?=w1341:bool)
        }
        n392 = local write "M2"(FALSE ("M2")) -> ()
        n393 = local write "M3"(TRUE ("M3")) -> ()
      }
    }
    n394 = case shown="True" w362 {
      frame False {
      }
      frame True {
        n395 = property on="estructura1" class="Bool (strict)"("Visible"=FALSE) -> ()  [unwired: 2 in, 2 out]
        n396 = property on="tarro vaciop" class="Bool (strict)"("Visible"=FALSE) -> ()  [unwired: 2 in, 2 out]
        n397 = property on="vastagoaux1" class="Bool (strict)"("Visible"=FALSE) -> ()  [unwired: 2 in, 2 out]
        n398 = property on="cuadroblanco" class="Bool (strict)"("Visible"=FALSE) -> ()  [unwired: 2 in, 2 out]
        n399 = while {
          stop <- w1331 stop-if-true
          n400 = property on="TARRO VACIO" class="Bool (strict)"() -> ("Top"=w1338:i32)  [unwired: 2 in, 2 out]
          n401 = Subtract(x=w1338, y=1) -> (x-y=w1336:i32)
          n402 = property on="TARRO VACIO" class="Bool (strict)"("Top"=w1336) -> ()  [unwired: 2 in, 2 out]
          n403 = Wait (ms)(milliseconds to wait=u32 0) -> ()  [unwired: 1 out]
          n404 = local read "RESET"() -> (w1332:bool)
          n405 = property on="TARRO VACIO" class="Bool (strict)"() -> ("Top"=w1335:i32)  [unwired: 2 in, 2 out]
          n406 = Less?(x=w1335, y=252) -> (x < y?=w1333:bool)
          n407 = Or(x=w1333, y=w1332) -> (x .or. y?=w1331:bool)
        }
        n408 = local write "M3"(FALSE ("M3")) -> ()
        n409 = local write "M4"(TRUE ("M4")) -> ()
      }
    }
    n410 = case shown="True" w352 {
      frame False {
      }
      frame True {
        n411 = property on="dep inferior" class="Bool (strict)"("Visible"=TRUE) -> ()  [unwired: 2 in, 2 out]
        n412 = property on="dep superior" class="Bool (strict)"("Visible"=FALSE) -> ()  [unwired: 2 in, 2 out]
        n413 = while {
          stop <- w1292 stop-if-true
          n414 = property on="PUERTA TOLVA" class="Bool (strict)"() -> ("Left"=w1303:i32)  [unwired: 2 in, 2 out]
          n415 = Subtract(x=w1303, y=1) -> (x-y=w1301:i32)
          n416 = property on="PUERTA TOLVA" class="Bool (strict)"("Left"=w1301) -> ()  [unwired: 2 in, 2 out]
          n417 = property on="perta tolva1" class="Bool (strict)"() -> ("Left"=w1297:i32)  [unwired: 2 in, 2 out]
          n418 = Add(x=w1297, y=1) -> (x+y=w1295:i32)
          n419 = property on="perta tolva1" class="Bool (strict)"("Left"=w1295) -> ()  [unwired: 2 in, 2 out]
          n420 = Wait (ms)(milliseconds to wait=u32 0) -> ()  [unwired: 1 out]
          n421 = local read "RESET"() -> (w1293:bool)
          n422 = property on="PUERTA TOLVA" class="Bool (strict)"() -> ("Left"=w1300:i32)  [unwired: 2 in, 2 out]
          n423 = Less?(x=w1300, y=930) -> (x < y?=w1298:bool)
          n424 = Or(x=w1298, y=w1293) -> (x .or. y?=w1292:bool)
        }
        n425 = local write "M5"(FALSE ("M5")) -> ()
        n426 = local write "M6"(TRUE ("M6")) -> ()
      }
    }
    n427 = case shown="True" w347 {
      frame False {
      }
      frame True {
        n428 = while {
          stop <- w1279 stop-if-true
          n429 = property on="puerta tolva2" class="Bool (strict)"() -> ("Left"=w1287:i32)  [unwired: 2 in, 2 out]
          n430 = Subtract(x=w1287, y=1) -> (x-y=w1285:i32)
          n431 = property on="puerta tolva2" class="Bool (strict)"("Left"=w1285) -> ()  [unwired: 2 in, 2 out]
          n432 = Wait (ms)(milliseconds to wait=u32 0) -> ()  [unwired: 1 out]
          n433 = local read "RESET"() -> (w1280:bool)
          n434 = property on="puerta tolva2" class="Bool (strict)"() -> ("Left"=w1284:i32)  [unwired: 2 in, 2 out]
          n435 = Less?(x=w1284, y=425) -> (x < y?=w1281:bool)
          n436 = Or(x=w1281, y=w1280) -> (x .or. y?=w1279:bool)
        }
        n437 = local write "M6"(FALSE ("M6")) -> ()
        n438 = local write "M7"(TRUE ("M7")) -> ()
      }
    }
    n439 = case shown="True" w342 {
      frame False {
      }
      frame True {
        n440 = property on="dep inferior" class="Bool (strict)"("Visible"=FALSE) -> ()  [unwired: 2 in, 2 out]
        n441 = property on="tarro llenop" class="Bool (strict)"("Visible"=TRUE) -> ()  [unwired: 2 in, 2 out]
        n442 = property on="tarro vaciop1" class="Bool (strict)"("Visible"=FALSE) -> ()  [unwired: 2 in, 2 out]
        n443 = while {
          stop <- w1268 stop-if-true
          n444 = property on="puerta tolva2" class="Bool (strict)"() -> ("Left"=w1276:i32)  [unwired: 2 in, 2 out]
          n445 = Add(x=w1276, y=1) -> (x+y=w1274:i32)
          n446 = property on="puerta tolva2" class="Bool (strict)"("Left"=w1274) -> ()  [unwired: 2 in, 2 out]
          n447 = Wait (ms)(milliseconds to wait=u32 0) -> ()  [unwired: 1 out]
          n448 = local read "RESET"() -> (w1269:bool)
          n449 = property on="puerta tolva2" class="Bool (strict)"() -> ("Left"=w1273:i32)  [unwired: 2 in, 2 out]
          n450 = Greater?(x=w1273, y=449) -> (0:w1270:bool)
          n451 = Or(x=w1270, y=w1269) -> (x .or. y?=w1268:bool)
        }
        n452 = local write "M7"(FALSE ("M7")) -> ()
        n453 = local write "M8"(TRUE ("M8")) -> ()
      }
    }
    n454 = case shown="True" w327 {
      frame False {
      }
      frame True {
        n455 = while {
          stop <- w1198 stop-if-true
          n456 = property on="vastago4 tapado" class="Bool (strict)"() -> ("Top"=w1206:i32)  [unwired: 2 in, 2 out]
          n457 = Add(x=w1206, y=1) -> (x+y=w1204:i32)
          n458 = property on="vastago4 tapado" class="Bool (strict)"("Top"=w1204) -> ()  [unwired: 2 in, 2 out]
          n459 = Wait (ms)(milliseconds to wait=u32 0) -> ()  [unwired: 1 out]
          n460 = local read "RESET"() -> (w1199:bool)
          n461 = property on="vastago4 tapado" class="Bool (strict)"() -> ("Top"=w1203:i32)  [unwired: 2 in, 2 out]
          n462 = Greater?(x=w1203, y=258) -> (0:w1200:bool)
          n463 = Or(x=w1200, y=w1199) -> (x .or. y?=w1198:bool)
        }
        n464 = local write "M10"(FALSE ("M10")) -> ()
        n465 = local write "M11"(TRUE ("M11")) -> ()
      }
    }
    n466 = case shown="True" w322 {
      frame False {
      }
      frame True {
        n467 = while {
          stop <- w1184 stop-if-true
          n468 = property on="tapa neutrop" class="Bool (strict)"() -> ("Top"=w1195:i32)  [unwired: 2 in, 2 out]
          n469 = Subtract(x=w1195, y=1) -> (x-y=w1193:i32)
          n470 = property on="tapa neutrop" class="Bool (strict)"("Top"=w1193) -> ()  [unwired: 2 in, 2 out]
          n471 = property on="vastago4 tapado" class="Bool (strict)"() -> ("Top"=w1192:i32)  [unwired: 2 in, 2 out]
          n472 = Subtract(x=w1192, y=1) -> (x-y=w1190:i32)
          n473 = property on="vastago4 tapado" class="Bool (strict)"("Top"=w1190) -> ()  [unwired: 2 in, 2 out]
          n474 = Wait (ms)(milliseconds to wait=u32 0) -> ()  [unwired: 1 out]
          n475 = local read "RESET"() -> (w1185:bool)
          n476 = property on="vastago4 tapado" class="Bool (strict)"() -> ("Top"=w1189:i32)  [unwired: 2 in, 2 out]
          n477 = Less?(x=w1189, y=227) -> (x < y?=w1186:bool)
          n478 = Or(x=w1186, y=w1185) -> (x .or. y?=w1184:bool)
        }
        n479 = local write "M11"(FALSE ("M11")) -> ()
        n480 = local write "M12"(TRUE ("M12")) -> ()
      }
    }
    n481 = case shown="True" w307 {
      frame False {
      }
      frame True {
        n482 = while {
          stop <- w1132 stop-if-true
          n483 = property on="vastago3 tapado" class="Bool (strict)"() -> ("Top"=w1143:i32)  [unwired: 2 in, 2 out]
          n484 = Subtract(x=w1143, y=1) -> (x-y=w1141:i32)
          n485 = property on="vastago3 tapado" class="Bool (strict)"("Top"=w1141) -> ()  [unwired: 2 in, 2 out]
          n486 = property on="vastago4 tapado" class="Bool (strict)"() -> ("Top"=w1140:i32)  [unwired: 2 in, 2 out]
          n487 = Subtract(x=w1140, y=2) -> (x-y=w1138:i32)
          n488 = property on="vastago4 tapado" class="Bool (strict)"("Top"=w1138) -> ()  [unwired: 2 in, 2 out]
          n489 = Wait (ms)(milliseconds to wait=u32 0) -> ()  [unwired: 1 out]
          n490 = local read "RESET"() -> (w1133:bool)
          n491 = property on="vastago3 tapado" class="Bool (strict)"() -> ("Top"=w1137:i32)  [unwired: 2 in, 2 out]
          n492 = Less?(x=w1137, y=207) -> (x < y?=w1134:bool)
          n493 = Or(x=w1134, y=w1133) -> (x .or. y?=w1132:bool)
        }
        n494 = local write "M14"(FALSE ("M14")) -> ()
        n495 = local write "M15"(TRUE ("M15")) -> ()
      }
    }
    n496 = case shown="True" w297 {
      frame False {
      }
      frame True {
        n497 = while {
          stop <- w1101 stop-if-true
          n498 = property on="BALANZA1" class="Bool (strict)"() -> ("Top"=w1109:i32)  [unwired: 2 in, 2 out]
          n499 = Subtract(x=w1109, y=2) -> (x-y=w1107:i32)
          n500 = property on="BALANZA1" class="Bool (strict)"("Top"=w1107) -> ()  [unwired: 2 in, 2 out]
          n501 = Wait (ms)(milliseconds to wait=u32 0) -> ()  [unwired: 1 out]
          n502 = local read "RESET"() -> (w1104:bool)
          n503 = property on="BALANZA1" class="Bool (strict)"() -> ("Top"=w1106:i32)  [unwired: 2 in, 2 out]
          n504 = Less?(x=w1106, y=109) -> (x < y?=w1103:bool)
          n505 = Or(x=w1103, y=w1104) -> (x .or. y?=w1101:bool)
        }
        n506 = local write "M16"(FALSE ("M16")) -> ()
        n507 = local write "M17"(TRUE ("M17")) -> ()
      }
    }
    n508 = case shown="True" w292 {
      frame False {
      }
      frame True {
        n509 = while {
          stop <- w1087 stop-if-true
          n510 = property on="BALANZA1" class="Bool (strict)"() -> ("Top"=w1098:i32)  [unwired: 2 in, 2 out]
          n511 = Subtract(x=w1098, y=2) -> (x-y=w1096:i32)
          n512 = property on="BALANZA1" class="Bool (strict)"("Top"=w1096) -> ()  [unwired: 2 in, 2 out]
          n513 = property on="TAPA NEUTRO" class="Bool (strict)"() -> ("Top"=w1092:i32)  [unwired: 2 in, 2 out]
          n514 = Subtract(x=w1092, y=2) -> (x-y=w1091:i32)
          n515 = property on="TAPA NEUTRO" class="Bool (strict)"("Top"=w1091) -> ()  [unwired: 2 in, 2 out]
          n516 = Wait (ms)(milliseconds to wait=u32 0) -> ()  [unwired: 1 out]
          n517 = local read "RESET"() -> (w1088:bool)
          n518 = property on="TAPA NEUTRO" class="Bool (strict)"() -> ("Top"=w1094:i32)  [unwired: 2 in, 2 out]
          n519 = Less?(x=w1094, y=16) -> (x < y?=w1090:bool)
          n520 = Or(x=w1090, y=w1088) -> (x .or. y?=w1087:bool)
        }
        n521 = local write "M17"(FALSE ("M17")) -> ()
        n522 = local write "M18"(TRUE ("M18")) -> ()
      }
    }
    n523 = case shown="True" w287 {
      frame False {
      }
      frame True {
        n524 = while {
          stop <- w1076 stop-if-true
          n525 = property on="BALANZA1" class="Bool (strict)"() -> ("Top"=w1084:i32)  [unwired: 2 in, 2 out]
          n526 = Add(x=w1084, y=2) -> (x+y=w1082:i32)
          n527 = property on="BALANZA1" class="Bool (strict)"("Top"=w1082) -> ()  [unwired: 2 in, 2 out]
          n528 = Wait (ms)(milliseconds to wait=u32 0) -> ()  [unwired: 1 out]
          n529 = local read "RESET"() -> (w1077:bool)
          n530 = property on="BALANZA1" class="Bool (strict)"() -> ("Top"=w1081:i32)  [unwired: 2 in, 2 out]
          n531 = Greater?(x=w1081, y=145) -> (0:w1078:bool)
          n532 = Or(x=w1078, y=w1077) -> (x .or. y?=w1076:bool)
        }
        n533 = local write "ANALIZANDO\nCC"(TRUE ("ANALIZANDO\nCC")) -> ()
        n534 = local write "M18"(FALSE ("M18")) -> ()
        n535 = local write "M19"(TRUE ("M19")) -> ()
      }
    }
    n536 = case shown="True" w279 {
      frame False {
      }
      frame True {
        n537 = while {
          stop <- w1038 stop-if-true
          n538 = property on="balanza2" class="Bool (strict)"() -> ("Left"=w1049:i32)  [unwired: 2 in, 2 out]
          n539 = Subtract(x=w1049, y=3) -> (x-y=w1047:i32)
          n540 = property on="balanza2" class="Bool (strict)"("Left"=w1047) -> ()  [unwired: 2 in, 2 out]
          n541 = property on="TAPA TARRO ROJO" class="Bool (strict)"() -> ("Left"=w1046:i32)  [unwired: 2 in, 2 out]
          n542 = Subtract(x=w1046, y=3) -> (x-y=w1044:i32)
          n543 = property on="TAPA TARRO ROJO" class="Bool (strict)"("Left"=w1044) -> ()  [unwired: 2 in, 2 out]
          n544 = Wait (ms)(milliseconds to wait=u32 0) -> ()  [unwired: 1 out]
          n545 = local read "RESET"() -> (w1039:bool)
          n546 = property on="balanza2" class="Bool (strict)"() -> ("Left"=w1042:i32)  [unwired: 2 in, 2 out]
          n547 = Less?(x=w1042, y=900) -> (x < y?=w1040:bool)
          n548 = Or(x=w1040, y=w1039) -> (x .or. y?=w1038:bool)
        }
        n549 = local write "M20"(FALSE ("M21")) -> ()
        n550 = local write "M21"(TRUE ("M22")) -> ()
      }
    }
    n551 = case shown="True" w274 {
      frame False {
      }
      frame True {
        n552 = while {
          stop <- w1024 stop-if-true
          n553 = property on="TAPA TARRO ROJO" class="Bool (strict)"() -> ("Left"=w1035:i32)  [unwired: 2 in, 2 out]
          n554 = Subtract(x=w1035, y=3) -> (x-y=w1033:i32)
          n555 = property on="TAPA TARRO ROJO" class="Bool (strict)"("Left"=w1033) -> ()  [unwired: 2 in, 2 out]
          n556 = property on="balanza2" class="Bool (strict)"() -> ("Left"=w1032:i32)  [unwired: 2 in, 2 out]
          n557 = Add(x=w1032, y=3) -> (x+y=w1030:i32)
          n558 = property on="balanza2" class="Bool (strict)"("Left"=w1030) -> ()  [unwired: 2 in, 2 out]
          n559 = Wait (ms)(milliseconds to wait=u32 0) -> ()  [unwired: 1 out]
          n560 = local read "RESET"() -> (w1025:bool)
          n561 = property on="balanza2" class="Bool (strict)"() -> ("Left"=w1028:i32)  [unwired: 2 in, 2 out]
          n562 = Greater?(x=w1028, y=977) -> (0:w1026:bool)
          n563 = Or(x=w1026, y=w1025) -> (x .or. y?=w1024:bool)
        }
        n564 = local write "M22"(TRUE ("M23")) -> ()
        n565 = local write "M21"(FALSE ("M22")) -> ()
      }
    }
    n566 = case shown="True" w269 {
      frame False {
      }
      frame True {
        n567 = while {
          stop <- w1013 stop-if-true
          n568 = property on="TAPA TARRO ROJO" class="Bool (strict)"() -> ("Left"=w1021:i32)  [unwired: 2 in, 2 out]
          n569 = Subtract(x=w1021, y=3) -> (x-y=w1019:i32)
          n570 = property on="TAPA TARRO ROJO" class="Bool (strict)"("Left"=w1019) -> ()  [unwired: 2 in, 2 out]
          n571 = Wait (ms)(milliseconds to wait=u32 0) -> ()  [unwired: 1 out]
          n572 = local read "RESET"() -> (w1014:bool)
          n573 = property on="TAPA TARRO ROJO" class="Bool (strict)"() -> ("Left"=w1017:i32)  [unwired: 2 in, 2 out]
          n574 = Less?(x=w1017, y=426) -> (x < y?=w1016:bool)
          n575 = Or(x=w1016, y=w1014) -> (x .or. y?=w1013:bool)
        }
        n576 = local write "M23"(TRUE ("M24")) -> ()
        n577 = local write "M22"(FALSE ("M23")) -> ()
      }
    }
    n578 = case shown="True" w264 {
      frame False {
      }
      frame True {
        n579 = while {
          stop <- w999 stop-if-true
          n580 = property on="VASTAGO MODULO6" class="Bool (strict)"() -> ("Top"=w1009:i32)  [unwired: 2 in, 2 out]
          n581 = Add(x=w1009, y=2) -> (x+y=w1007:i32)
          n582 = property on="VASTAGO MODULO6" class="Bool (strict)"("Top"=w1007) -> ()  [unwired: 2 in, 2 out]
          n583 = property on="TAPA TARRO ROJO" class="Bool (strict)"() -> ("Top"=w1006:i32)  [unwired: 2 in, 2 out]
          n584 = Add(x=w1006, y=2) -> (x+y=w1004:i32)
          n585 = property on="TAPA TARRO ROJO" class="Bool (strict)"("Top"=w1004) -> ()  [unwired: 2 in, 2 out]
          n586 = Wait (ms)(milliseconds to wait=u32 0) -> ()  [unwired: 1 out]
          n587 = local read "RESET"() -> (w1000:bool)
          n588 = property on="VASTAGO MODULO6" class="Bool (strict)"() -> ("Top"=w1003:i32)  [unwired: 2 in, 2 out]
          n589 = Greater?(x=w1003, y=55) -> (0:w1002:bool)
          n590 = Or(x=w1002, y=w1000) -> (x .or. y?=w999:bool)
        }
        n591 = local write "M23"(FALSE ("M24")) -> ()
        n592 = local write "M24"(TRUE ("M25")) -> ()
        n593 = Wait (ms)(milliseconds to wait=u32 1000) -> ()  [unwired: 1 out]
      }
    }
    n594 = case shown="True" w259 {
      frame False {
      }
      frame True {
        n595 = local read "FINALIZADOS\nROJOS"() -> (w986:dbl)
        n596 = Increment(x=w986) -> (x+1=w985:dbl)
        n597 = local write "FINALIZADOS\nROJOS"(w985) -> ()
        n598 = while {
          stop <- w987 stop-if-true
          n599 = property on="VASTAGO MODULO6" class="Bool (strict)"() -> ("Top"=w995:i32)  [unwired: 2 in, 2 out]
          n600 = Subtract(x=w995, y=1) -> (x-y=w993:i32)
          n601 = property on="VASTAGO MODULO6" class="Bool (strict)"("Top"=w993) -> ()  [unwired: 2 in, 2 out]
          n602 = Wait (ms)(milliseconds to wait=u32 0) -> ()  [unwired: 1 out]
          n603 = local read "RESET"() -> (w988:bool)
          n604 = property on="VASTAGO MODULO6" class="Bool (strict)"() -> ("Top"=w991:i32)  [unwired: 2 in, 2 out]
          n605 = Less?(x=w991, y=-10) -> (x < y?=w989:bool)
          n606 = Or(x=w989, y=w988) -> (x .or. y?=w987:bool)
        }
        n607 = local write "M25"(TRUE ("M30")) -> ()
        n608 = local write "M24"(FALSE ("M25")) -> ()
        n609 = local write "PESO\nSI"(FALSE ("PESO\nSI")) -> ()
        n610 = local write "ROJO"(FALSE ("ROJO")) -> ()
      }
    }
    n611 = case shown="True" w254 {
      frame False {
      }
      frame True {
        n612 = property on="TAPA TARRO ROJO" class="Bool (strict)"("Visible"=FALSE) -> ()  [unwired: 2 in, 2 out]
        n613 = local write "M25"(FALSE ("M30")) -> ()
      }
    }
    n614 = case shown="True" w242 {
      frame False {
      }
      frame True {
        n615 = while {
          stop <- w944 stop-if-true
          n616 = property on="TAPA AZUL" class="Bool (strict)"() -> ("Left"=w955:i32)  [unwired: 2 in, 2 out]
          n617 = Subtract(x=w955, y=3) -> (x-y=w953:i32)
          n618 = property on="TAPA AZUL" class="Bool (strict)"("Left"=w953) -> ()  [unwired: 2 in, 2 out]
          n619 = property on="balanza2" class="Bool (strict)"() -> ("Left"=w952:i32)  [unwired: 2 in, 2 out]
          n620 = Subtract(x=w952, y=3) -> (x-y=w950:i32)
          n621 = property on="balanza2" class="Bool (strict)"("Left"=w950) -> ()  [unwired: 2 in, 2 out]
          n622 = Wait (ms)(milliseconds to wait=u32 0) -> ()  [unwired: 1 out]
          n623 = local read "RESET"() -> (w945:bool)
          n624 = property on="balanza2" class="Bool (strict)"() -> ("Left"=w948:i32)  [unwired: 2 in, 2 out]
          n625 = Less?(x=w948, y=900) -> (x < y?=w946:bool)
          n626 = Or(x=w946, y=w945) -> (x .or. y?=w944:bool)
        }
        n627 = local write "M26"(FALSE ("M26")) -> ()
        n628 = local write "M27"(TRUE ("M27")) -> ()
      }
    }
    n629 = case shown="True" w237 {
      frame False {
      }
      frame True {
        n630 = while {
          stop <- w930 stop-if-true
          n631 = property on="balanza2" class="Bool (strict)"() -> ("Left"=w940:i32)  [unwired: 2 in, 2 out]
          n632 = Add(x=w940, y=3) -> (x+y=w941:i32)
          n633 = property on="balanza2" class="Bool (strict)"("Left"=w941) -> ()  [unwired: 2 in, 2 out]
          n634 = property on="TAPA AZUL" class="Bool (strict)"() -> ("Left"=w937:i32)  [unwired: 2 in, 2 out]
          n635 = Subtract(x=w937, y=3) -> (x-y=w938:i32)
          n636 = property on="TAPA AZUL" class="Bool (strict)"("Left"=w938) -> ()  [unwired: 2 in, 2 out]
          n637 = Wait (ms)(milliseconds to wait=u32 0) -> ()  [unwired: 1 out]
          n638 = local read "RESET"() -> (w931:bool)
          n639 = property on="balanza2" class="Bool (strict)"() -> ("Left"=w934:i32)  [unwired: 2 in, 2 out]
          n640 = Greater?(x=w934, y=977) -> (0:w932:bool)
          n641 = Or(x=w932, y=w931) -> (x .or. y?=w930:bool)
        }
        n642 = local write "M28"(TRUE ("M28")) -> ()
        n643 = local write "M27"(FALSE ("M27")) -> ()
      }
    }
    n644 = case shown="True" w232 {
      frame False {
      }
      frame True {
        n645 = while {
          stop <- w919 stop-if-true
          n646 = property on="TAPA AZUL" class="Bool (strict)"() -> ("Left"=w927:i32)  [unwired: 2 in, 2 out]
          n647 = Subtract(x=w927, y=3) -> (x-y=w925:i32)
          n648 = property on="TAPA AZUL" class="Bool (strict)"("Left"=w925) -> ()  [unwired: 2 in, 2 out]
          n649 = Wait (ms)(milliseconds to wait=u32 0) -> ()  [unwired: 1 out]
          n650 = local read "RESET"() -> (w920:bool)
          n651 = property on="TAPA AZUL" class="Bool (strict)"() -> ("Left"=w923:i32)  [unwired: 2 in, 2 out]
          n652 = Less?(x=w923, y=426) -> (x < y?=w921:bool)
          n653 = Or(x=w921, y=w920) -> (x .or. y?=w919:bool)
        }
        n654 = local write "M28"(FALSE ("M28")) -> ()
        n655 = local write "M29"(TRUE ("M29")) -> ()
      }
    }
    n656 = case shown="True" w222 {
      frame False {
      }
      frame True {
        n657 = while {
          stop <- w885 stop-if-true
          n658 = property on="TAPA AZUL" class="Bool (strict)"() -> ("Top"=w896:i32)  [unwired: 2 in, 2 out]
          n659 = Add(x=w896, y=2) -> (x+y=w894:i32)
          n660 = property on="TAPA AZUL" class="Bool (strict)"("Top"=w894) -> ()  [unwired: 2 in, 2 out]
          n661 = property on="VASTAGO MODULO6" class="Bool (strict)"() -> ("Top"=w893:i32)  [unwired: 2 in, 2 out]
          n662 = Add(x=w893, y=2) -> (x+y=w891:i32)
          n663 = property on="VASTAGO MODULO6" class="Bool (strict)"("Top"=w891) -> ()  [unwired: 2 in, 2 out]
          n664 = Wait (ms)(milliseconds to wait=u32 0) -> ()  [unwired: 1 out]
          n665 = local read "RESET"() -> (w886:bool)
          n666 = property on="VASTAGO MODULO6" class="Bool (strict)"() -> ("Top"=w889:i32)  [unwired: 2 in, 2 out]
          n667 = Greater?(x=w889, y=55) -> (0:w887:bool)
          n668 = Or(x=w887, y=w886) -> (x .or. y?=w885:bool)
        }
        n669 = local write "M30"(FALSE ("M30")) -> ()
        n670 = local write "M31"(TRUE ("M31")) -> ()
      }
    }
    n671 = case shown="True" w207 {
      frame False {
      }
      frame True {
        n672 = property on="TAPA AZUL" class="Bool (strict)"("Visible"=FALSE) -> ()  [unwired: 2 in, 2 out]
        n673 = local write "M33"(FALSE ("M33")) -> ()
      }
    }
    n674 = case shown="True" w198 {
      frame False {
      }
      frame True {
        n675 = while {
          stop <- w808 stop-if-true
          n676 = property on="TAPA NOCOLOR" class="Bool (strict)"() -> ("Left"=w819:i32)  [unwired: 2 in, 2 out]
          n677 = Subtract(x=w819, y=6) -> (x-y=w817:i32)
          n678 = property on="TAPA NOCOLOR" class="Bool (strict)"("Left"=w817) -> ()  [unwired: 2 in, 2 out]
          n679 = property on="balanza2" class="Bool (strict)"() -> ("Left"=w816:i32)  [unwired: 2 in, 2 out]
          n680 = Subtract(x=w816, y=6) -> (x-y=w814:i32)
          n681 = property on="balanza2" class="Bool (strict)"("Left"=w814) -> ()  [unwired: 2 in, 2 out]
          n682 = Wait (ms)(milliseconds to wait=u32 0) -> ()  [unwired: 1 out]
          n683 = local read "RESET"() -> (w809:bool)
          n684 = property on="balanza2" class="Bool (strict)"() -> ("Left"=w812:i32)  [unwired: 2 in, 2 out]
          n685 = Less?(x=w812, y=900) -> (x < y?=w810:bool)
          n686 = Or(x=w810, y=w809) -> (x .or. y?=w808:bool)
        }
        n687 = local write "M34"(FALSE ("M34")) -> ()
        n688 = local write "M35"(TRUE ("M35")) -> ()
      }
    }
    n689 = case shown="True" w193 {
      frame False {
      }
      frame True {
        n690 = while {
          stop <- w794 stop-if-true
          n691 = property on="balanza2" class="Bool (strict)"() -> ("Left"=w804:i32)  [unwired: 2 in, 2 out]
          n692 = Add(x=w804, y=6) -> (x+y=w805:i32)
          n693 = property on="balanza2" class="Bool (strict)"("Left"=w805) -> ()  [unwired: 2 in, 2 out]
          n694 = property on="TAPA NOCOLOR" class="Bool (strict)"() -> ("Left"=w802:i32)  [unwired: 2 in, 2 out]
          n695 = Subtract(x=w802, y=6) -> (x-y=w800:i32)
          n696 = property on="TAPA NOCOLOR" class="Bool (strict)"("Left"=w800) -> ()  [unwired: 2 in, 2 out]
          n697 = Wait (ms)(milliseconds to wait=u32 0) -> ()  [unwired: 1 out]
          n698 = local read "RESET"() -> (w795:bool)
          n699 = property on="balanza2" class="Bool (strict)"() -> ("Left"=w798:i32)  [unwired: 2 in, 2 out]
          n700 = Greater?(x=w798, y=977) -> (0:w796:bool)
          n701 = Or(x=w796, y=w795) -> (x .or. y?=w794:bool)
        }
        n702 = local write "M35"(FALSE ("M35")) -> ()
        n703 = local write "M36"(TRUE ("M36")) -> ()
      }
    }
    n704 = case shown="True" w186 {
      frame False {
      }
      frame True {
        n705 = while {
          stop <- w783 stop-if-true
          n706 = property on="TAPA NOCOLOR" class="Bool (strict)"() -> ("Left"=w791:i32)  [unwired: 2 in, 2 out]
          n707 = Subtract(x=w791, y=6) -> (x-y=w789:i32)
          n708 = property on="TAPA NOCOLOR" class="Bool (strict)"("Left"=w789) -> ()  [unwired: 2 in, 2 out]
          n709 = Wait (ms)(milliseconds to wait=u32 0) -> ()  [unwired: 1 out]
          n710 = local read "RESET"() -> (w784:bool)
          n711 = property on="TAPA NOCOLOR" class="Bool (strict)"() -> ("Left"=w787:i32)  [unwired: 2 in, 2 out]
          n712 = Less?(x=w787, y=737) -> (x < y?=w785:bool)
          n713 = Or(x=w785, y=w784) -> (x .or. y?=w783:bool)
        }
        n714 = local write "M37"(TRUE ("M37")) -> ()
        n715 = local write "M36"(FALSE ("M36")) -> ()
      }
    }
    n716 = case shown="True" w151 {
      frame False {
      }
      frame True {
        n717 = property on="PINZA ABIERTA" class="Bool (strict)"("Visible"=FALSE) -> ()  [unwired: 2 in, 2 out]
        n718 = property on="VASTAGO RECHAZO" class="Bool (strict)"("Visible"=FALSE) -> ()  [unwired: 2 in, 2 out]
        n719 = local write "M43"(FALSE ("M43")) -> ()
        n720 = property on="TARRO NOCOLOR" class="Bool (strict)"("Visible"=FALSE) -> ()  [unwired: 2 in, 2 out]
        n721 = property on="CILINDRO RECHAZO" class="Bool (strict)"("Visible"=FALSE) -> ()  [unwired: 2 in, 2 out]
        n722 = property on="CILINDRO RECHAZO1" class="Bool (strict)"("Visible"=FALSE) -> ()  [unwired: 2 in, 2 out]
        n723 = property on="TAPA NOCOLOR" class="Bool (strict)"("Visible"=FALSE) -> ()  [unwired: 2 in, 2 out]
        n724 = property on="ESTRUCTURA RECHAZO" class="Bool (strict)"("Visible"=FALSE) -> ()  [unwired: 2 in, 2 out]
        n725 = property on="DEPOSITO NOCOLOR" class="Bool (strict)"("Visible"=FALSE) -> ()  [unwired: 2 in, 2 out]
        n726 = property on="DEPOSITO NOPESO" class="Bool (strict)"("Visible"=FALSE) -> ()  [unwired: 2 in, 2 out]
      }
    }
    n727 = case shown="True" w136 {
      frame False {
      }
      frame True {
        n728 = while {
          stop <- w584 stop-if-true
          n729 = property on="TAPA NOPESO" class="Bool (strict)"() -> ("Left"=w595:i32)  [unwired: 2 in, 2 out]
          n730 = Subtract(x=w595, y=6) -> (x-y=w593:i32)
          n731 = property on="TAPA NOPESO" class="Bool (strict)"("Left"=w593) -> ()  [unwired: 2 in, 2 out]
          n732 = property on="balanza2" class="Bool (strict)"() -> ("Left"=w592:i32)  [unwired: 2 in, 2 out]
          n733 = Subtract(x=w592, y=6) -> (x-y=w590:i32)
          n734 = property on="balanza2" class="Bool (strict)"("Left"=w590) -> ()  [unwired: 2 in, 2 out]
          n735 = Wait (ms)(milliseconds to wait=u32 0) -> ()  [unwired: 1 out]
          n736 = local read "RESET"() -> (w585:bool)
          n737 = property on="balanza2" class="Bool (strict)"() -> ("Left"=w588:i32)  [unwired: 2 in, 2 out]
          n738 = Less?(x=w588, y=900) -> (x < y?=w586:bool)
          n739 = Or(x=w586, y=w585) -> (x .or. y?=w584:bool)
        }
        n740 = local write "M44"(FALSE ("M44")) -> ()
        n741 = local write "M45"(TRUE ("M45")) -> ()
      }
    }
    n742 = case shown="True" w131 {
      frame False {
      }
      frame True {
        n743 = while {
          stop <- w570 stop-if-true
          n744 = property on="TAPA NOPESO" class="Bool (strict)"() -> ("Left"=w581:i32)  [unwired: 2 in, 2 out]
          n745 = Subtract(x=w581, y=6) -> (x-y=w579:i32)
          n746 = property on="TAPA NOPESO" class="Bool (strict)"("Left"=w579) -> ()  [unwired: 2 in, 2 out]
          n747 = property on="balanza2" class="Bool (strict)"() -> ("Left"=w578:i32)  [unwired: 2 in, 2 out]
          n748 = Add(x=w578, y=6) -> (x+y=w576:i32)
          n749 = property on="balanza2" class="Bool (strict)"("Left"=w576) -> ()  [unwired: 2 in, 2 out]
          n750 = Wait (ms)(milliseconds to wait=u32 0) -> ()  [unwired: 1 out]
          n751 = local read "RESET"() -> (w571:bool)
          n752 = property on="balanza2" class="Bool (strict)"() -> ("Left"=w574:i32)  [unwired: 2 in, 2 out]
          n753 = Greater?(x=w574, y=977) -> (0:w572:bool)
          n754 = Or(x=w572, y=w571) -> (x .or. y?=w570:bool)
        }
        n755 = local write "M45"(FALSE ("M45")) -> ()
        n756 = local write "M46"(TRUE ("M46")) -> ()
      }
    }
    n757 = case shown="True" w126 {
      frame False {
      }
      frame True {
        n758 = while {
          stop <- w559 stop-if-true
          n759 = property on="TAPA NOPESO" class="Bool (strict)"() -> ("Left"=w567:i32)  [unwired: 2 in, 2 out]
          n760 = Subtract(x=w567, y=6) -> (x-y=w565:i32)
          n761 = property on="TAPA NOPESO" class="Bool (strict)"("Left"=w565) -> ()  [unwired: 2 in, 2 out]
          n762 = Wait (ms)(milliseconds to wait=u32 0) -> ()  [unwired: 1 out]
          n763 = local read "RESET"() -> (w560:bool)
          n764 = property on="TAPA NOPESO" class="Bool (strict)"() -> ("Left"=w563:i32)  [unwired: 2 in, 2 out]
          n765 = Less?(x=w563, y=737) -> (x < y?=w561:bool)
          n766 = Or(x=w561, y=w560) -> (x .or. y?=w559:bool)
        }
        n767 = local write "M46"(FALSE ("M46")) -> ()
        n768 = local write "M47"(TRUE ("M47")) -> ()
      }
    }
    n769 = case shown="True" w89 {
      frame False {
      }
      frame True {
        n770 = property on="PINZA ABIERTA" class="Bool (strict)"("Visible"=FALSE) -> ()  [unwired: 2 in, 2 out]
        n771 = property on="VASTAGO RECHAZO" class="Bool (strict)"("Visible"=FALSE) -> ()  [unwired: 2 in, 2 out]
        n772 = property on="TAPA NOPESO" class="Bool (strict)"("Visible"=FALSE) -> ()  [unwired: 2 in, 2 out]
        n773 = property on="CILINDRO RECHAZO" class="Bool (strict)"("Visible"=FALSE) -> ()  [unwired: 2 in, 2 out]
        n774 = property on="CILINDRO RECHAZO1" class="Bool (strict)"("Visible"=FALSE) -> ()  [unwired: 2 in, 2 out]
        n775 = property on="TARRO NOPESO" class="Bool (strict)"("Visible"=FALSE) -> ()  [unwired: 2 in, 2 out]
        n776 = property on="ESTRUCTURA RECHAZO" class="Bool (strict)"("Visible"=FALSE) -> ()  [unwired: 2 in, 2 out]
        n777 = property on="DEPOSITO NOPESO" class="Bool (strict)"("Visible"=FALSE) -> ()  [unwired: 2 in, 2 out]
        n778 = property on="DEPOSITO NOCOLOR" class="Bool (strict)"("Visible"=FALSE) -> ()  [unwired: 2 in, 2 out]
        n779 = local write "M54"(FALSE ("M54")) -> ()
      }
    }
    n780 = case shown="True" w202 {
      frame False {
      }
      frame True {
        n781 = property on="TAPA NEUTRO" class="Bool (strict)"("Visible"=FALSE) -> ()  [unwired: 2 in, 2 out]
        n782 = property on="TAPA NOCOLOR" class="Bool (strict)"("Visible"=TRUE) -> ()  [unwired: 2 in, 2 out]
        n783 = property on="ACTUADOR RECHAZO" class="Bool (strict)"("Top"=220 ("Position:Top")) -> ()  [unwired: 2 in, 2 out]
        n784 = property on="VASTAGO RECHAZO" class="Bool (strict)"("Top"=180 ("Position:Top")) -> ()  [unwired: 2 in, 2 out]
        n785 = property on="CILINDRO RECHAZO" class="Bool (strict)"("Left"=592 ("Position:Left")) -> ()  [unwired: 2 in, 2 out]
        n786 = property on="CILINDRO RECHAZO1" class="Bool (strict)"("Left"=620 ("Position:Left")) -> ()  [unwired: 2 in, 2 out]
        n787 = property on="VASTAGO RECHAZO" class="Bool (strict)"("Left"=614 ("Position:Left")) -> ()  [unwired: 2 in, 2 out]
        n788 = property on="TAPA NOCOLOR" class="Bool (strict)"("Top"=14 ("Position:Top")) -> ()  [unwired: 2 in, 2 out]
        n789 = property on="TAPA NOCOLOR" class="Bool (strict)"("Left"=917 ("Position:Left")) -> ()  [unwired: 2 in, 2 out]
        n790 = property on="PINZA CERRADA" class="Bool (strict)"("Top"=316 ("Position:Top")) -> ()  [unwired: 2 in, 2 out]
        n791 = property on="PINZA CERRADA" class="Bool (strict)"("Left"=596 ("Position:Left")) -> ()  [unwired: 2 in, 2 out]
        n792 = property on="PINZA ABIERTA" class="Bool (strict)"("Left"=587 ("Position:Left")) -> ()  [unwired: 2 in, 2 out]
        n793 = property on="PINZA ABIERTA" class="Bool (strict)"("Top"=313 ("Position:Top")) -> ()  [unwired: 2 in, 2 out]
        n794 = property on="TARRO NOCOLOR" class="Bool (strict)"("Top"=409 ("Position:Top")) -> ()  [unwired: 2 in, 2 out]
        n795 = property on="TARRO NOCOLOR" class="Bool (strict)"("Left"=386 ("Position:Left")) -> ()  [unwired: 2 in, 2 out]
        n796 = local write "reinicio"(TRUE ("reinicio")) -> ()
        n797 = while {
          stop <- w840 stop-if-true
          n798 = property on="balanza2" class="Bool (strict)"() -> ("Left"=w848:i32)  [unwired: 2 in, 2 out]
          n799 = Subtract(x=w848, y=6) -> (x-y=w846:i32)
          n800 = property on="balanza2" class="Bool (strict)"("Left"=w846) -> ()  [unwired: 2 in, 2 out]
          n801 = Wait (ms)(milliseconds to wait=u32 0) -> ()  [unwired: 1 out]
          n802 = local read "RESET"() -> (w841:bool)
          n803 = property on="balanza2" class="Bool (strict)"() -> ("Left"=w844:i32)  [unwired: 2 in, 2 out]
          n804 = Less?(x=w844, y=965) -> (x < y?=w842:bool)
          n805 = Or(x=w842, y=w841) -> (x .or. y?=w840:bool)
        }
        n806 = local write "ANALIZANDO\nCC"(FALSE ("ANALIZANDO\nCC")) -> ()
        n807 = local write "NO \nCOLOR"(TRUE ("NO \nCOLOR")) -> ()
        n808 = local write "M19"(FALSE ("M19")) -> ()
        n809 = local write "M34"(TRUE ("M34")) -> ()
      }
    }
    n810 = case shown="True" w357 {
      frame False {
      }
      frame True {
        n811 = property on="cilindros tolva" class="Bool (strict)"("Visible"=TRUE) -> ()  [unwired: 2 in, 2 out]
        n812 = property on="perta tolva1" class="Bool (strict)"("Visible"=TRUE) -> ()  [unwired: 2 in, 2 out]
        n813 = property on="tarro vaciop1" class="Bool (strict)"("Visible"=TRUE) -> ()  [unwired: 2 in, 2 out]
        n814 = property on="dep superior" class="Bool (strict)"("Visible"=TRUE) -> ()  [unwired: 2 in, 2 out]
        n815 = property on="puerta tolva2" class="Bool (strict)"("Visible"=TRUE) -> ()  [unwired: 2 in, 2 out]
        n816 = property on="tolva vacia" class="Bool (strict)"("Visible"=TRUE) -> ()  [unwired: 2 in, 2 out]
        n817 = while {
          stop <- w1312 stop-if-true
          n818 = property on="PUERTA TOLVA" class="Bool (strict)"() -> ("Left"=w1323:i32)  [unwired: 2 in, 2 out]
          n819 = Add(x=w1323, y=1) -> (x+y=w1321:i32)
          n820 = property on="PUERTA TOLVA" class="Bool (strict)"("Left"=w1321) -> ()  [unwired: 2 in, 2 out]
          n821 = property on="perta tolva1" class="Bool (strict)"() -> ("Left"=w1317:i32)  [unwired: 2 in, 2 out]
          n822 = Subtract(x=w1317, y=1) -> (x-y=w1315:i32)
          n823 = property on="perta tolva1" class="Bool (strict)"("Left"=w1315) -> ()  [unwired: 2 in, 2 out]
          n824 = Wait (ms)(milliseconds to wait=u32 0) -> ()  [unwired: 1 out]
          n825 = property on="PUERTA TOLVA" class="Bool (strict)"() -> ("Left"=w1320:i32)  [unwired: 2 in, 2 out]
          n826 = local read "RESET"() -> (w1313:bool)
          n827 = Greater?(x=w1320, y=950) -> (0:w1318:bool)
          n828 = Or(x=w1318, y=w1313) -> (x .or. y?=w1312:bool)
        }
        n829 = local write "M4"(FALSE ("M4")) -> ()
        n830 = local write "M5"(TRUE ("M5")) -> ()
      }
    }
    n831 = case shown="True" w337 {
      frame False {
      }
      frame True {
        n832 = property on="TARRO VACIO" class="Bool (strict)"("Visible"=FALSE) -> ()  [unwired: 2 in, 2 out]
        n833 = property on="CAJA LLENA" class="Bool (strict)"("Visible"=TRUE) -> ()  [unwired: 2 in, 2 out]
        n834 = property on="tarro vaciop1" class="Bool (strict)"("Visible"=FALSE) -> ()  [unwired: 2 in, 2 out]
        n835 = property on="tolva vacia" class="Bool (strict)"("Visible"=FALSE) -> ()  [unwired: 2 in, 2 out]
        n836 = property on="dep inferior" class="Bool (strict)"("Visible"=FALSE) -> ()  [unwired: 2 in, 2 out]
        n837 = property on="dep superior" class="Bool (strict)"("Visible"=FALSE) -> ()  [unwired: 2 in, 2 out]
        n838 = property on="cilindros tolva" class="Bool (strict)"("Visible"=FALSE) -> ()  [unwired: 2 in, 2 out]
        n839 = property on="puerta tolva2" class="Bool (strict)"("Visible"=FALSE) -> ()  [unwired: 2 in, 2 out]
        n840 = property on="perta tolva1" class="Bool (strict)"("Visible"=FALSE) -> ()  [unwired: 2 in, 2 out]
        n841 = property on="tarro llenop" class="Bool (strict)"("Visible"=FALSE) -> ()  [unwired: 2 in, 2 out]
        n842 = while {
          stop <- w1255 stop-if-true
          n843 = property on="CAJA LLENA" class="Bool (strict)"() -> ("Top"=w1262:i32)  [unwired: 2 in, 2 out]
          n844 = Subtract(x=w1262, y=2) -> (x-y=w1260:i32)
          n845 = property on="CAJA LLENA" class="Bool (strict)"("Top"=w1260) -> ()  [unwired: 2 in, 2 out]
          n846 = Wait (ms)(milliseconds to wait=u32 0) -> ()  [unwired: 1 out]
          n847 = local read "RESET"() -> (w1256:bool)
          n848 = property on="CAJA LLENA" class="Bool (strict)"() -> ("Top"=w1259:i32)  [unwired: 2 in, 2 out]
          n849 = Less?(x=w1259, y=97) -> (x < y?=w1257:bool)
          n850 = Or(x=w1257, y=w1256) -> (x .or. y?=w1255:bool)
        }
        n851 = local write "M8"(FALSE ("M8")) -> ()
        n852 = local write "M9"(TRUE ("M9")) -> ()
      }
    }
    n853 = case shown="True" w312 {
      frame False {
      }
      frame True {
        n854 = while {
          stop <- w1146 stop-if-true
          n855 = property on="tapa neutrop" class="Bool (strict)"() -> ("Top"=w1160:i32)  [unwired: 2 in, 2 out]
          n856 = Add(x=w1160, y=2) -> (x+y=w1158:i32)
          n857 = property on="tapa neutrop" class="Bool (strict)"("Top"=w1158) -> ()  [unwired: 2 in, 2 out]
          n858 = property on="vastago3 tapado" class="Bool (strict)"() -> ("Top"=w1157:i32)  [unwired: 2 in, 2 out]
          n859 = Add(x=w1157, y=1) -> (x+y=w1155:i32)
          n860 = property on="vastago3 tapado" class="Bool (strict)"("Top"=w1155) -> ()  [unwired: 2 in, 2 out]
          n861 = property on="vastago4 tapado" class="Bool (strict)"() -> ("Top"=w1154:i32)  [unwired: 2 in, 2 out]
          n862 = Add(x=w1154, y=2) -> (x+y=w1152:i32)
          n863 = property on="vastago4 tapado" class="Bool (strict)"("Top"=w1152) -> ()  [unwired: 2 in, 2 out]
          n864 = Wait (ms)(milliseconds to wait=u32 0) -> ()  [unwired: 1 out]
          n865 = local read "RESET"() -> (w1147:bool)
          n866 = property on="tapa neutrop" class="Bool (strict)"() -> ("Top"=w1151:i32)  [unwired: 2 in, 2 out]
          n867 = Greater?(x=w1151, y=367) -> (0:w1148:bool)
          n868 = Or(x=w1148, y=w1147) -> (x .or. y?=w1146:bool)
        }
        n869 = local write "M13"(FALSE ("M13")) -> ()
        n870 = local write "M14"(TRUE ("M14")) -> ()
      }
    }
    n871 = case shown="True" w302 {
      frame False {
      }
      frame True {
        n872 = property on="estructura tapado" class="Bool (strict)"("Visible"=FALSE) -> ()  [unwired: 2 in, 2 out]
        n873 = property on="tapa neutrop" class="Bool (strict)"("Visible"=FALSE) -> ()  [unwired: 2 in, 2 out]
        n874 = property on="vastago1 tapado" class="Bool (strict)"("Visible"=FALSE) -> ()  [unwired: 2 in, 2 out]
        n875 = property on="cilindro1 tapado" class="Bool (strict)"("Visible"=FALSE) -> ()  [unwired: 2 in, 2 out]
        n876 = property on="vastago2 tapado" class="Bool (strict)"("Visible"=FALSE) -> ()  [unwired: 2 in, 2 out]
        n877 = property on="cilindro2 tapado" class="Bool (strict)"("Visible"=FALSE) -> ()  [unwired: 2 in, 2 out]
        n878 = property on="vastago3 tapado" class="Bool (strict)"("Visible"=FALSE) -> ()  [unwired: 2 in, 2 out]
        n879 = property on="cilindro3 tapado" class="Bool (strict)"("Visible"=FALSE) -> ()  [unwired: 2 in, 2 out]
        n880 = property on="vastago4 tapado" class="Bool (strict)"("Visible"=FALSE) -> ()  [unwired: 2 in, 2 out]
        n881 = while {
          stop <- w1121 stop-if-true
          n882 = property on="TAPA NEUTRO" class="Bool (strict)"() -> ("Top"=w1129:i32)  [unwired: 2 in, 2 out]
          n883 = Subtract(x=w1129, y=1) -> (x-y=w1127:i32)
          n884 = property on="TAPA NEUTRO" class="Bool (strict)"("Top"=w1127) -> ()  [unwired: 2 in, 2 out]
          n885 = Wait (ms)(milliseconds to wait=u32 0) -> ()  [unwired: 1 out]
          n886 = local read "RESET"() -> (w1123:bool)
          n887 = property on="TAPA NEUTRO" class="Bool (strict)"() -> ("Top"=w1126:i32)  [unwired: 2 in, 2 out]
          n888 = Less?(x=w1126, y=67) -> (x < y?=w1124:bool)
          n889 = Or(x=w1124, y=w1123) -> (x .or. y?=w1121:bool)
        }
        n890 = local write "M15"(FALSE ("M15")) -> ()
        n891 = local write "M16"(TRUE ("M16")) -> ()
      }
    }
    n892 = case shown="True" w282 {
      frame False {
      }
      frame True {
        n893 = property on="TAPA NEUTRO" class="Bool (strict)"("Visible"=FALSE) -> ()  [unwired: 2 in, 2 out]
        n894 = property on="TAPA TARRO ROJO" class="Bool (strict)"("Visible"=TRUE) -> ()  [unwired: 2 in, 2 out]
        n895 = property on="TAPA TARRO ROJO" class="Bool (strict)"("Left"=916 ("Position:Left")) -> ()  [unwired: 2 in, 2 out]
        n896 = property on="TAPA TARRO ROJO" class="Bool (strict)"("Top"=14 ("Position:Top")) -> ()  [unwired: 2 in, 2 out]
        n897 = property on="CILINDRO MODULO6" class="Bool (strict)"("Left"=376 ("Position:Left")) -> ()  [unwired: 2 in, 2 out]
        n898 = property on="VASTAGO MODULO6" class="Bool (strict)"("Left"=385 ("Position:Left")) -> ()  [unwired: 2 in, 2 out]
        n899 = property on="VASTAGO MODULO6" class="Bool (strict)"("Top"=-11 ("Position:Top")) -> ()  [unwired: 2 in, 2 out]
        n900 = property on="MODULO6" class="Bool (strict)"("Left"=378 ("Position:Left")) -> ()  [unwired: 2 in, 2 out]
        n901 = local write "reinicio"(TRUE ("reinicio")) -> ()
        n902 = while {
          stop <- w1067 stop-if-true
          n903 = property on="balanza2" class="Bool (strict)"() -> ("Left"=w1072:i32)  [unwired: 2 in, 2 out]
          n904 = Subtract(x=w1072, y=3) -> (x-y=w1070:i32)
          n905 = property on="balanza2" class="Bool (strict)"("Left"=w1070) -> ()  [unwired: 2 in, 2 out]
          n906 = Wait (ms)(milliseconds to wait=u32 0) -> ()  [unwired: 1 out]
          n907 = local read "RESET"() -> (w1065:bool)
          n908 = property on="balanza2" class="Bool (strict)"() -> ("Left"=w1069:i32)  [unwired: 2 in, 2 out]
          n909 = Less?(x=w1069, y=965) -> (x < y?=w1066:bool)
          n910 = Or(x=w1066, y=w1065) -> (x .or. y?=w1067:bool)
        }
        n911 = local write "ANALIZANDO\nCC"(FALSE ("ANALIZANDO\nCC")) -> ()
        n912 = local write "M19"(FALSE ("M20")) -> ()
        n913 = local write "M20"(TRUE ("M21")) -> ()
        n914 = local write "PESO\nSI"(TRUE ("PESO\nSI")) -> ()
        n915 = local write "ROJO"(TRUE ("ROJO")) -> ()
      }
    }
    n916 = case shown="True" w247 {
      frame False {
      }
      frame True {
        n917 = property on="TAPA NEUTRO" class="Bool (strict)"("Visible"=FALSE) -> ()  [unwired: 2 in, 2 out]
        n918 = property on="TAPA AZUL" class="Bool (strict)"("Visible"=TRUE) -> ()  [unwired: 2 in, 2 out]
        n919 = property on="TAPA AZUL" class="Bool (strict)"("Top"=14 ("Position:Top")) -> ()  [unwired: 2 in, 2 out]
        n920 = property on="TAPA AZUL" class="Bool (strict)"("Left"=917 ("Position:Left")) -> ()  [unwired: 2 in, 2 out]
        n921 = property on="VASTAGO MODULO6" class="Bool (strict)"("Top"=-11 ("Position:Top")) -> ()  [unwired: 2 in, 2 out]
        n922 = property on="MODULO6" class="Bool (strict)"("Left"=378 ("Position:Left")) -> ()  [unwired: 2 in, 2 out]
        n923 = property on="CILINDRO MODULO6" class="Bool (strict)"("Left"=376 ("Position:Left")) -> ()  [unwired: 2 in, 2 out]
        n924 = property on="VASTAGO MODULO6" class="Bool (strict)"("Left"=385 ("Position:Left")) -> ()  [unwired: 2 in, 2 out]
        n925 = local write "reinicio"(TRUE ("reinicio")) -> ()
        n926 = while {
          stop <- w971 stop-if-true
          n927 = property on="balanza2" class="Bool (strict)"() -> ("Left"=w977:i32)  [unwired: 2 in, 2 out]
          n928 = Subtract(x=w977, y=3) -> (x-y=w978:i32)
          n929 = property on="balanza2" class="Bool (strict)"("Left"=w978) -> ()  [unwired: 2 in, 2 out]
          n930 = Wait (ms)(milliseconds to wait=u32 0) -> ()  [unwired: 1 out]
          n931 = local read "RESET"() -> (w970:bool)
          n932 = property on="balanza2" class="Bool (strict)"() -> ("Left"=w974:i32)  [unwired: 2 in, 2 out]
          n933 = Less?(x=w974, y=965) -> (x < y?=w972:bool)
          n934 = Or(x=w972, y=w970) -> (x .or. y?=w971:bool)
        }
        n935 = local write "ANALIZANDO\nCC"(FALSE ("ANALIZANDO\nCC")) -> ()
        n936 = local write "AZUL"(TRUE ("AZUL")) -> ()
        n937 = local write "M19"(FALSE ("M19")) -> ()
        n938 = local write "PESO\nSI"(TRUE ("PESO\nSI")) -> ()
        n939 = local write "M26"(TRUE ("M26")) -> ()
      }
    }
    n940 = case shown="True" w227 {
      frame False {
      }
      frame True {
        n941 = while {
          stop <- w899 stop-if-true
          n942 = property on="TAPA AZUL" class="Bool (strict)"() -> ("Left"=w916:i32)  [unwired: 2 in, 2 out]
          n943 = Subtract(x=w916, y=2) -> (x-y=w914:i32)
          n944 = property on="TAPA AZUL" class="Bool (strict)"("Left"=w914) -> ()  [unwired: 2 in, 2 out]
          n945 = property on="CILINDRO MODULO6" class="Bool (strict)"() -> ("Left"=w913:i32)  [unwired: 2 in, 2 out]
          n946 = Subtract(x=w913, y=2) -> (x-y=w911:i32)
          n947 = property on="CILINDRO MODULO6" class="Bool (strict)"("Left"=w911) -> ()  [unwired: 2 in, 2 out]
          n948 = property on="VASTAGO MODULO6" class="Bool (strict)"() -> ("Left"=w910:i32)  [unwired: 2 in, 2 out]
          n949 = Subtract(x=w910, y=2) -> (x-y=w908:i32)
          n950 = property on="VASTAGO MODULO6" class="Bool (strict)"("Left"=w908) -> ()  [unwired: 2 in, 2 out]
          n951 = property on="MODULO6" class="Bool (strict)"() -> ("Left"=w907:i32)  [unwired: 2 in, 2 out]
          n952 = Subtract(x=w907, y=2) -> (x-y=w905:i32)
          n953 = property on="MODULO6" class="Bool (strict)"("Left"=w905) -> ()  [unwired: 2 in, 2 out]
          n954 = Wait (ms)(milliseconds to wait=u32 0) -> ()  [unwired: 1 out]
          n955 = local read "RESET"() -> (w901:bool)
          n956 = property on="MODULO6" class="Bool (strict)"() -> ("Left"=w904:i32)  [unwired: 2 in, 2 out]
          n957 = Less?(x=w904, y=316) -> (x < y?=w902:bool)
          n958 = Or(x=w902, y=w901) -> (x .or. y?=w899:bool)
        }
        n959 = local write "M29"(FALSE ("M29")) -> ()
        n960 = local write "M30"(TRUE ("M30")) -> ()
      }
    }
    n961 = case shown="True" w212 {
      frame False {
      }
      frame True {
        n962 = while {
          stop <- w853 stop-if-true
          n963 = property on="CILINDRO MODULO6" class="Bool (strict)"() -> ("Left"=w867:i32)  [unwired: 2 in, 2 out]
          n964 = Add(x=w867, y=3) -> (x+y=w865:i32)
          n965 = property on="CILINDRO MODULO6" class="Bool (strict)"("Left"=w865) -> ()  [unwired: 2 in, 2 out]
          n966 = property on="VASTAGO MODULO6" class="Bool (strict)"() -> ("Left"=w864:i32)  [unwired: 2 in, 2 out]
          n967 = Add(x=w864, y=3) -> (x+y=w862:i32)
          n968 = property on="VASTAGO MODULO6" class="Bool (strict)"("Left"=w862) -> ()  [unwired: 2 in, 2 out]
          n969 = property on="MODULO6" class="Bool (strict)"() -> ("Left"=w861:i32)  [unwired: 2 in, 2 out]
          n970 = Add(x=w861, y=3) -> (x+y=w859:i32)
          n971 = property on="MODULO6" class="Bool (strict)"("Left"=w859) -> ()  [unwired: 2 in, 2 out]
          n972 = Wait (ms)(milliseconds to wait=u32 0) -> ()  [unwired: 1 out]
          n973 = local read "RESET"() -> (w854:bool)
          n974 = property on="MODULO6" class="Bool (strict)"() -> ("Left"=w857:i32)  [unwired: 2 in, 2 out]
          n975 = Greater?(x=w857, y=377) -> (0:w855:bool)
          n976 = Or(x=w855, y=w854) -> (x .or. y?=w853:bool)
        }
        n977 = local write "M32"(FALSE ("M32")) -> ()
        n978 = local write "M33"(TRUE ("M33")) -> ()
      }
    }
    n979 = case shown="True" w176 {
      frame False {
      }
      frame True {
        n980 = while {
          stop <- w732 stop-if-true
          n981 = property on="VASTAGO RECHAZO" class="Bool (strict)"() -> ("Top"=w746:i32)  [unwired: 2 in, 2 out]
          n982 = Add(x=w746, y=6) -> (x+y=w744:i32)
          n983 = property on="VASTAGO RECHAZO" class="Bool (strict)"("Top"=w744) -> ()  [unwired: 2 in, 2 out]
          n984 = property on="PINZA ABIERTA" class="Bool (strict)"() -> ("Top"=w743:i32)  [unwired: 2 in, 2 out]
          n985 = Add(x=w743, y=6) -> (x+y=w741:i32)
          n986 = property on="PINZA ABIERTA" class="Bool (strict)"("Top"=w741) -> ()  [unwired: 2 in, 2 out]
          n987 = property on="PINZA CERRADA" class="Bool (strict)"() -> ("Top"=w740:i32)  [unwired: 2 in, 2 out]
          n988 = Add(x=w740, y=6) -> (x+y=w738:i32)
          n989 = property on="PINZA CERRADA" class="Bool (strict)"("Top"=w738) -> ()  [unwired: 2 in, 2 out]
          n990 = Wait (ms)(milliseconds to wait=u32 0) -> ()  [unwired: 1 out]
          n991 = local read "RESET"() -> (w733:bool)
          n992 = property on="PINZA CERRADA" class="Bool (strict)"() -> ("Top"=w736:i32)  [unwired: 2 in, 2 out]
          n993 = Greater?(x=w736, y=396) -> (0:w734:bool)
          n994 = Or(x=w734, y=w733) -> (x .or. y?=w732:bool)
        }
        n995 = local write "M38"(FALSE ("M38")) -> ()
        n996 = local write "M39"(TRUE ("M39")) -> ()
      }
    }
    n997 = case shown="True" w161 {
      frame False {
      }
      frame True {
        n998 = while {
          stop <- w659 stop-if-true
          n999 = property on="PINZA ABIERTA" class="Bool (strict)"() -> ("Top"=w676:i32)  [unwired: 2 in, 2 out]
          n1000 = Add(x=w676, y=6) -> (x+y=w674:i32)
          n1001 = property on="PINZA ABIERTA" class="Bool (strict)"("Top"=w674) -> ()  [unwired: 2 in, 2 out]
          n1002 = property on="VASTAGO RECHAZO" class="Bool (strict)"() -> ("Top"=w673:i32)  [unwired: 2 in, 2 out]
          n1003 = Add(x=w673, y=6) -> (x+y=w671:i32)
          n1004 = property on="VASTAGO RECHAZO" class="Bool (strict)"("Top"=w671) -> ()  [unwired: 2 in, 2 out]
          n1005 = property on="TARRO NOCOLOR" class="Bool (strict)"() -> ("Top"=w670:i32)  [unwired: 2 in, 2 out]
          n1006 = Add(x=w670, y=6) -> (x+y=w668:i32)
          n1007 = property on="TARRO NOCOLOR" class="Bool (strict)"("Top"=w668) -> ()  [unwired: 2 in, 2 out]
          n1008 = property on="PINZA CERRADA" class="Bool (strict)"() -> ("Top"=w667:i32)  [unwired: 2 in, 2 out]
          n1009 = Add(x=w667, y=6) -> (x+y=w665:i32)
          n1010 = property on="PINZA CERRADA" class="Bool (strict)"("Top"=w665) -> ()  [unwired: 2 in, 2 out]
          n1011 = Wait (ms)(milliseconds to wait=u32 0) -> ()  [unwired: 1 out]
          n1012 = local read "RESET"() -> (w660:bool)
          n1013 = property on="PINZA CERRADA" class="Bool (strict)"() -> ("Top"=w663:i32)  [unwired: 2 in, 2 out]
          n1014 = Greater?(x=w663, y=396) -> (0:w661:bool)
          n1015 = Or(x=w661, y=w660) -> (x .or. y?=w659:bool)
        }
        n1016 = local write "M41"(FALSE ("M41")) -> ()
        n1017 = local write "M42"(TRUE ("M42")) -> ()
      }
    }
    n1018 = case shown="True" w119 {
      frame False {
      }
      frame True {
        n1019 = while {
          stop <- w508 stop-if-true
          n1020 = property on="VASTAGO RECHAZO" class="Bool (strict)"() -> ("Top"=w522:i32)  [unwired: 2 in, 2 out]
          n1021 = Add(x=w522, y=6) -> (x+y=w520:i32)
          n1022 = property on="VASTAGO RECHAZO" class="Bool (strict)"("Top"=w520) -> ()  [unwired: 2 in, 2 out]
          n1023 = property on="PINZA ABIERTA" class="Bool (strict)"() -> ("Top"=w519:i32)  [unwired: 2 in, 2 out]
          n1024 = Add(x=w519, y=6) -> (x+y=w517:i32)
          n1025 = property on="PINZA ABIERTA" class="Bool (strict)"("Top"=w517) -> ()  [unwired: 2 in, 2 out]
          n1026 = property on="PINZA CERRADA" class="Bool (strict)"() -> ("Top"=w516:i32)  [unwired: 2 in, 2 out]
          n1027 = Add(x=w516, y=6) -> (x+y=w514:i32)
          n1028 = property on="PINZA CERRADA" class="Bool (strict)"("Top"=w514) -> ()  [unwired: 2 in, 2 out]
          n1029 = Wait (ms)(milliseconds to wait=u32 0) -> ()  [unwired: 1 out]
          n1030 = local read "RESET"() -> (w509:bool)
          n1031 = property on="PINZA CERRADA" class="Bool (strict)"() -> ("Top"=w512:i32)  [unwired: 2 in, 2 out]
          n1032 = Greater?(x=w512, y=396) -> (0:w510:bool)
          n1033 = Or(x=w510, y=w509) -> (x .or. y?=w508:bool)
        }
        n1034 = local write "M48"(FALSE ("M48")) -> ()
        n1035 = local write "M49"(TRUE ("M49")) -> ()
      }
    }
    n1036 = case shown="True" w104 {
      frame False {
      }
      frame True {
        n1037 = while {
          stop <- w434 stop-if-true
          n1038 = property on="PINZA ABIERTA" class="Bool (strict)"() -> ("Top"=w451:i32)  [unwired: 2 in, 2 out]
          n1039 = Add(x=w451, y=6) -> (x+y=w449:i32)
          n1040 = property on="PINZA ABIERTA" class="Bool (strict)"("Top"=w449) -> ()  [unwired: 2 in, 2 out]
          n1041 = property on="VASTAGO RECHAZO" class="Bool (strict)"() -> ("Top"=w448:i32)  [unwired: 2 in, 2 out]
          n1042 = Add(x=w448, y=6) -> (x+y=w446:i32)
          n1043 = property on="VASTAGO RECHAZO" class="Bool (strict)"("Top"=w446) -> ()  [unwired: 2 in, 2 out]
          n1044 = property on="TARRO NOPESO" class="Bool (strict)"() -> ("Top"=w445:i32)  [unwired: 2 in, 2 out]
          n1045 = Add(x=w445, y=6) -> (x+y=w443:i32)
          n1046 = property on="TARRO NOPESO" class="Bool (strict)"("Top"=w443) -> ()  [unwired: 2 in, 2 out]
          n1047 = property on="PINZA CERRADA" class="Bool (strict)"() -> ("Top"=w442:i32)  [unwired: 2 in, 2 out]
          n1048 = Add(x=w442, y=6) -> (x+y=w440:i32)
          n1049 = property on="PINZA CERRADA" class="Bool (strict)"("Top"=w440) -> ()  [unwired: 2 in, 2 out]
          n1050 = Wait (ms)(milliseconds to wait=u32 0) -> ()  [unwired: 1 out]
          n1051 = local read "RESET"() -> (w435:bool)
          n1052 = property on="PINZA CERRADA" class="Bool (strict)"() -> ("Top"=w438:i32)  [unwired: 2 in, 2 out]
          n1053 = Greater?(x=w438, y=396) -> (0:w436:bool)
          n1054 = Or(x=w436, y=w435) -> (x .or. y?=w434:bool)
        }
        n1055 = local write "M51"(FALSE ("M51")) -> ()
        n1056 = local write "M52"(TRUE ("M52")) -> ()
      }
    }
    n1057 = Not(x=w80) -> (.not. x?=w68:bool)
    n1058 = Not(x=w81) -> (.not. x?=w64:bool)
    n1059 = Not(x=w77) -> (.not. x?=w65:bool)
    n1060 = Not(x=w78) -> (.not. x?=w66:bool)
    n1061 = case shown="True" w317 {
      frame False {
      }
      frame True {
        n1062 = property on="CAJA LLENA" class="Bool (strict)"("Visible"=FALSE) -> ()  [unwired: 2 in, 2 out]
        n1063 = while {
          stop <- w1165 stop-if-true
          n1064 = property on="CILINDRO NUEVO" class="Bool (strict)"() -> ("Left"=w1181:i32)  [unwired: 2 in, 2 out]
          n1065 = Subtract(x=w1181, y=1) -> (x-y=w1179:i32)
          n1066 = property on="CILINDRO NUEVO" class="Bool (strict)"("Left"=w1179) -> ()  [unwired: 2 in, 2 out]
          n1067 = property on="BASTAGO TAPAS" class="Bool (strict)"() -> ("Left"=w1176:i32)  [unwired: 2 in, 2 out]
          n1068 = Add(x=w1176, y=3) -> (x+y=w1174:i32)
          n1069 = property on="BASTAGO TAPAS" class="Bool (strict)"("Left"=w1174) -> ()  [unwired: 2 in, 2 out]
          n1070 = property on="vastago1 tapado" class="Bool (strict)"() -> ("Left"=w1172:i32)  [unwired: 2 in, 2 out]
          n1071 = Subtract(x=w1172, y=3) -> (x-y=w1170:i32)
          n1072 = property on="vastago1 tapado" class="Bool (strict)"("Left"=w1170) -> ()  [unwired: 2 in, 2 out]
          n1073 = property on="vastago2 tapado" class="Bool (strict)"() -> ("Left"=w1169:i32)  [unwired: 2 in, 2 out]
          n1074 = Add(x=w1169, y=1) -> (x+y=w1167:i32)
          n1075 = property on="vastago2 tapado" class="Bool (strict)"("Left"=w1167) -> ()  [unwired: 2 in, 2 out]
          n1076 = Wait (ms)(milliseconds to wait=u32 0) -> ()  [unwired: 1 out]
          n1077 = local read "RESET"() -> (w1164:bool)
          n1078 = property on="CILINDRO NUEVO" class="Bool (strict)"() -> ("Left"=w1178:i32)  [unwired: 2 in, 2 out]
          n1079 = Less?(x=w1178, y=870) -> (x < y?=w1173:bool)
          n1080 = Or(x=w1173, y=w1164) -> (x .or. y?=w1165:bool)
        }
        n1081 = local write "M12"(FALSE ("M12")) -> ()
        n1082 = local write "M13"(TRUE ("M13")) -> ()
      }
    }
    n1083 = case shown="True" w171 {
      frame False {
      }
      frame True {
        n1084 = property on="PINZA CERRADA" class="Bool (strict)"("Visible"=TRUE) -> ()  [unwired: 2 in, 2 out]
        n1085 = property on="PINZA ABIERTA" class="Bool (strict)"("Visible"=FALSE) -> ()  [unwired: 2 in, 2 out]
        n1086 = while {
          stop <- w713 stop-if-true
          n1087 = property on="PINZA ABIERTA" class="Bool (strict)"() -> ("Top"=w729:i32)  [unwired: 2 in, 2 out]
          n1088 = Subtract(x=w729, y=6) -> (x-y=w727:i32)
          n1089 = property on="PINZA ABIERTA" class="Bool (strict)"("Top"=w727) -> ()  [unwired: 2 in, 2 out]
          n1090 = property on="VASTAGO RECHAZO" class="Bool (strict)"() -> ("Top"=w726:i32)  [unwired: 2 in, 2 out]
          n1091 = Subtract(x=w726, y=6) -> (x-y=w724:i32)
          n1092 = property on="VASTAGO RECHAZO" class="Bool (strict)"("Top"=w724) -> ()  [unwired: 2 in, 2 out]
          n1093 = property on="TARRO NOCOLOR" class="Bool (strict)"() -> ("Top"=w723:i32)  [unwired: 2 in, 2 out]
          n1094 = Subtract(x=w723, y=6) -> (x-y=w721:i32)
          n1095 = property on="TARRO NOCOLOR" class="Bool (strict)"("Top"=w721) -> ()  [unwired: 2 in, 2 out]
          n1096 = property on="PINZA CERRADA" class="Bool (strict)"() -> ("Top"=w720:i32)  [unwired: 2 in, 2 out]
          n1097 = Subtract(x=w720, y=6) -> (x-y=w718:i32)
          n1098 = property on="PINZA CERRADA" class="Bool (strict)"("Top"=w718) -> ()  [unwired: 2 in, 2 out]
          n1099 = local read "RESET"() -> (w714:bool)
          n1100 = property on="PINZA CERRADA" class="Bool (strict)"() -> ("Top"=w717:i32)  [unwired: 2 in, 2 out]
          n1101 = Less?(x=w717, y=317) -> (x < y?=w715:bool)
          n1102 = Or(x=w715, y=w714) -> (x .or. y?=w713:bool)
        }
        n1103 = local write "M40"(TRUE ("M40")) -> ()
        n1104 = local write "M39"(FALSE ("M39")) -> ()
      }
    }
    n1105 = case shown="True" w146 {
      frame False {
      }
      frame True {
        n1106 = property on="TAPA NEUTRO" class="Bool (strict)"("Visible"=FALSE) -> ()  [unwired: 2 in, 2 out]
        n1107 = property on="TAPA NOPESO" class="Bool (strict)"("Visible"=TRUE) -> ()  [unwired: 2 in, 2 out]
        n1108 = property on="ACTUADOR RECHAZO" class="Bool (strict)"("Top"=220 ("Position:Top")) -> ()  [unwired: 2 in, 2 out]
        n1109 = property on="VASTAGO RECHAZO" class="Bool (strict)"("Top"=180 ("Position:Top")) -> ()  [unwired: 2 in, 2 out]
        n1110 = property on="CILINDRO RECHAZO" class="Bool (strict)"("Left"=592 ("Position:Left")) -> ()  [unwired: 2 in, 2 out]
        n1111 = property on="CILINDRO RECHAZO1" class="Bool (strict)"("Left"=620 ("Position:Left")) -> ()  [unwired: 2 in, 2 out]
        n1112 = property on="VASTAGO RECHAZO" class="Bool (strict)"("Left"=614 ("Position:Left")) -> ()  [unwired: 2 in, 2 out]
        n1113 = property on="TAPA NOPESO" class="Bool (strict)"("Top"=14 ("Position:Top")) -> ()  [unwired: 2 in, 2 out]
        n1114 = property on="TAPA NOPESO" class="Bool (strict)"("Left"=917 ("Position:Left")) -> ()  [unwired: 2 in, 2 out]
        n1115 = property on="PINZA CERRADA" class="Bool (strict)"("Top"=316 ("Position:Top")) -> ()  [unwired: 2 in, 2 out]
        n1116 = property on="PINZA CERRADA" class="Bool (strict)"("Left"=596 ("Position:Left")) -> ()  [unwired: 2 in, 2 out]
        n1117 = property on="PINZA ABIERTA" class="Bool (strict)"("Left"=587 ("Position:Left")) -> ()  [unwired: 2 in, 2 out]
        n1118 = property on="PINZA ABIERTA" class="Bool (strict)"("Top"=313 ("Position:Top")) -> ()  [unwired: 2 in, 2 out]
        n1119 = property on="TARRO NOPESO" class="Bool (strict)"("Top"=409 ("Position:Top")) -> ()  [unwired: 2 in, 2 out]
        n1120 = property on="TARRO NOPESO" class="Bool (strict)"("Left"=386 ("Position:Left")) -> ()  [unwired: 2 in, 2 out]
        n1121 = local write "reinicio"(TRUE ("reinicio")) -> ()
        n1122 = while {
          stop <- w616 stop-if-true
          n1123 = property on="balanza2" class="Bool (strict)"() -> ("Left"=w624:i32)  [unwired: 2 in, 2 out]
          n1124 = Subtract(x=w624, y=6) -> (x-y=w622:i32)
          n1125 = property on="balanza2" class="Bool (strict)"("Left"=w622) -> ()  [unwired: 2 in, 2 out]
          n1126 = Wait (ms)(milliseconds to wait=u32 0) -> ()  [unwired: 1 out]
          n1127 = local read "RESET"() -> (w617:bool)
          n1128 = property on="balanza2" class="Bool (strict)"() -> ("Left"=w621:i32)  [unwired: 2 in, 2 out]
          n1129 = Less?(x=w621, y=965) -> (x < y?=w618:bool)
          n1130 = Or(x=w618, y=w617) -> (x .or. y?=w616:bool)
        }
        n1131 = local write "ANALIZANDO\nCC"(FALSE ("ANALIZANDO\nCC")) -> ()
        n1132 = local write "PESO\nNO"(TRUE ("PESO\nNO")) -> ()
        n1133 = local write "M19"(FALSE ("M19")) -> ()
        n1134 = local write "M44"(TRUE ("M44")) -> ()
      }
    }
    n1135 = case shown="True" w114 {
      frame False {
      }
      frame True {
        n1136 = property on="PINZA ABIERTA" class="Bool (strict)"("Visible"=FALSE) -> ()  [unwired: 2 in, 2 out]
        n1137 = property on="PINZA CERRADA" class="Bool (strict)"("Visible"=TRUE) -> ()  [unwired: 2 in, 2 out]
        n1138 = while {
          stop <- w488 stop-if-true
          n1139 = property on="PINZA ABIERTA" class="Bool (strict)"() -> ("Top"=w505:i32)  [unwired: 2 in, 2 out]
          n1140 = Subtract(x=w505, y=6) -> (x-y=w503:i32)
          n1141 = property on="PINZA ABIERTA" class="Bool (strict)"("Top"=w503) -> ()  [unwired: 2 in, 2 out]
          n1142 = property on="VASTAGO RECHAZO" class="Bool (strict)"() -> ("Top"=w502:i32)  [unwired: 2 in, 2 out]
          n1143 = Subtract(x=w502, y=6) -> (x-y=w500:i32)
          n1144 = property on="VASTAGO RECHAZO" class="Bool (strict)"("Top"=w500) -> ()  [unwired: 2 in, 2 out]
          n1145 = property on="TARRO NOPESO" class="Bool (strict)"() -> ("Top"=w499:i32)  [unwired: 2 in, 2 out]
          n1146 = Subtract(x=w499, y=6) -> (x-y=w497:i32)
          n1147 = property on="TARRO NOPESO" class="Bool (strict)"("Top"=w497) -> ()  [unwired: 2 in, 2 out]
          n1148 = property on="PINZA CERRADA" class="Bool (strict)"() -> ("Top"=w496:i32)  [unwired: 2 in, 2 out]
          n1149 = Subtract(x=w496, y=6) -> (x-y=w494:i32)
          n1150 = property on="PINZA CERRADA" class="Bool (strict)"("Top"=w494) -> ()  [unwired: 2 in, 2 out]
          n1151 = Wait (ms)(milliseconds to wait=u32 0) -> ()  [unwired: 1 out]
          n1152 = local read "RESET"() -> (w489:bool)
          n1153 = property on="PINZA CERRADA" class="Bool (strict)"() -> ("Top"=w492:i32)  [unwired: 2 in, 2 out]
          n1154 = Less?(x=w492, y=317) -> (x < y?=w490:bool)
          n1155 = Or(x=w490, y=w489) -> (x .or. y?=w488:bool)
        }
        n1156 = local write "M49"(FALSE ("M49")) -> ()
        n1157 = local write "M50"(TRUE ("M50")) -> ()
      }
    }
    n1158 = Not(x=w79) -> (.not. x?=w67:bool)
    n1159 = case shown="True" w62 {
      frame False {
      }
      frame True {
        n1160 = property on="TARRO VACIO" class="Bool (strict)"("Top"=412 ("Position:Top")) -> ()  [unwired: 2 in, 2 out]
        n1161 = property on="CAJA LLENA" class="Bool (strict)"("Top"=250 ("Position:Top")) -> ()  [unwired: 2 in, 2 out]
        n1162 = property on="BALANZA1" class="Bool (strict)"("Top"=146 ("Position:Top")) -> ()  [unwired: 2 in, 2 out]
        n1163 = property on="PUERTA TOLVA" class="Bool (strict)"("Left"=929 ("Position:Left")) -> ()  [unwired: 2 in, 2 out]
        n1164 = property on="CILINDRO NUEVO" class="Bool (strict)"("Left"=869 ("Position:Left")) -> ()  [unwired: 2 in, 2 out]
        n1165 = property on="TAPA NEUTRO" class="Bool (strict)"("Top"=96 ("Position:Top")) -> ()  [unwired: 2 in, 2 out]
        n1166 = property on="TARRO VACIO" class="Bool (strict)"("Visible"=FALSE) -> ()  [unwired: 2 in, 2 out]
        n1167 = property on="TAPA NEUTRO" class="Bool (strict)"("Left"=980 ("Position:Left")) -> ()  [unwired: 2 in, 2 out]
        n1168 = property on="TAPA NEUTRO" class="Bool (strict)"("Visible"=FALSE) -> ()  [unwired: 2 in, 2 out]
        n1169 = property on="TARRO NOPESO" class="Bool (strict)"("Visible"=FALSE) -> ()  [unwired: 2 in, 2 out]
        n1170 = property on="estructura1" class="Bool (strict)"("Visible"=FALSE) -> ()  [unwired: 2 in, 2 out]
        n1171 = property on="TAPA NOPESO" class="Bool (strict)"("Visible"=FALSE) -> ()  [unwired: 2 in, 2 out]
        n1172 = property on="tarro vaciop" class="Bool (strict)"("Visible"=FALSE) -> ()  [unwired: 2 in, 2 out]
        n1173 = property on="vastagoaux1" class="Bool (strict)"("Visible"=FALSE) -> ()  [unwired: 2 in, 2 out]
        n1174 = property on="cuadroblanco" class="Bool (strict)"("Visible"=FALSE) -> ()  [unwired: 2 in, 2 out]
        n1175 = property on="TAPA TARRO ROJO" class="Bool (strict)"("Visible"=FALSE) -> ()  [unwired: 2 in, 2 out]
        n1176 = property on="VASTAGO MODULO6" class="Bool (strict)"("Top"=-11 ("Position:Top")) -> ()  [unwired: 2 in, 2 out]
        n1177 = property on="TAPA AZUL" class="Bool (strict)"("Top"=14 ("Position:Top")) -> ()  [unwired: 2 in, 2 out]
        n1178 = property on="VASTAGO MODULO6" class="Bool (strict)"("Left"=385 ("Position:Left")) -> ()  [unwired: 2 in, 2 out]
        n1179 = property on="TAPA AZUL" class="Bool (strict)"("Left"=917 ("Position:Left")) -> ()  [unwired: 2 in, 2 out]
        n1180 = property on="TAPA AZUL" class="Bool (strict)"("Visible"=FALSE) -> ()  [unwired: 2 in, 2 out]
        n1181 = property on="MODULO6" class="Bool (strict)"("Left"=378 ("Position:Left")) -> ()  [unwired: 2 in, 2 out]
        n1182 = property on="CILINDRO MODULO6" class="Bool (strict)"("Left"=376 ("Position:Left")) -> ()  [unwired: 2 in, 2 out]
        n1183 = property on="CAJA LLENA" class="Bool (strict)"("Visible"=FALSE) -> ()  [unwired: 2 in, 2 out]
        n1184 = property on="dep inferior" class="Bool (strict)"("Visible"=FALSE) -> ()  [unwired: 2 in, 2 out]
        n1185 = property on="dep superior" class="Bool (strict)"("Visible"=FALSE) -> ()  [unwired: 2 in, 2 out]
        n1186 = property on="cilindros tolva" class="Bool (strict)"("Visible"=FALSE) -> ()  [unwired: 2 in, 2 out]
        n1187 = property on="puerta tolva2" class="Bool (strict)"("Visible"=FALSE) -> ()  [unwired: 2 in, 2 out]
        n1188 = property on="perta tolva1" class="Bool (strict)"("Visible"=FALSE) -> ()  [unwired: 2 in, 2 out]
        n1189 = property on="vastagoaux1" class="Bool (strict)"("Top"=420 ("Position:Top")) -> ()  [unwired: 2 in, 2 out]
        n1190 = property on="BASTAGO TAPAS" class="Bool (strict)"("Left"=973 ("Position:Left")) -> ()  [unwired: 2 in, 2 out]
        n1191 = property on="tarro vaciop" class="Bool (strict)"("Top"=358 ("Position:Top")) -> ()  [unwired: 2 in, 2 out]
        n1192 = property on="tapa neutrop" class="Bool (strict)"("Top"=345 ("Position:Top")) -> ()  [unwired: 2 in, 2 out]
        n1193 = property on="tapa neutrop" class="Bool (strict)"("Left"=527 ("Position:Left")) -> ()  [unwired: 2 in, 2 out]
        n1194 = property on="vastago1 tapado" class="Bool (strict)"("Left"=361 ("Position:Left")) -> ()  [unwired: 2 in, 2 out]
        n1195 = property on="balanza2" class="Bool (strict)"("Left"=978 ("Position:Left")) -> ()  [unwired: 2 in, 2 out]
        n1196 = property on="PINZA ABIERTA" class="Bool (strict)"("Visible"=FALSE) -> ()  [unwired: 2 in, 2 out]
        n1197 = property on="VASTAGO RECHAZO" class="Bool (strict)"("Visible"=FALSE) -> ()  [unwired: 2 in, 2 out]
        n1198 = property on="ACTUADOR RECHAZO" class="Bool (strict)"("Top"=220 ("Position:Top")) -> ()  [unwired: 2 in, 2 out]
        n1199 = property on="TAPA NOCOLOR" class="Bool (strict)"("Top"=14 ("Position:Top")) -> ()  [unwired: 2 in, 2 out]
        n1200 = property on="TARRO NOCOLOR" class="Bool (strict)"("Visible"=FALSE) -> ()  [unwired: 2 in, 2 out]
        n1201 = property on="TAPA NOCOLOR" class="Bool (strict)"("Left"=917 ("Position:Left")) -> ()  [unwired: 2 in, 2 out]
        n1202 = property on="PINZA ABIERTA" class="Bool (strict)"("Top"=313 ("Position:Top")) -> ()  [unwired: 2 in, 2 out]
        n1203 = property on="TARRO NOCOLOR" class="Bool (strict)"("Left"=386 ("Position:Left")) -> ()  [unwired: 2 in, 2 out]
        n1204 = property on="PINZA ABIERTA" class="Bool (strict)"("Left"=587 ("Position:Left")) -> ()  [unwired: 2 in, 2 out]
        n1205 = property on="tolva vacia" class="Bool (strict)"("Visible"=FALSE) -> ()  [unwired: 2 in, 2 out]
        n1206 = property on="tarro vaciop1" class="Bool (strict)"("Visible"=FALSE) -> ()  [unwired: 2 in, 2 out]
        n1207 = property on="tarro llenop" class="Bool (strict)"("Visible"=FALSE) -> ()  [unwired: 2 in, 2 out]
        n1208 = property on="estructura tapado" class="Bool (strict)"("Visible"=FALSE) -> ()  [unwired: 2 in, 2 out]
        n1209 = property on="tapa neutrop" class="Bool (strict)"("Visible"=FALSE) -> ()  [unwired: 2 in, 2 out]
        n1210 = property on="vastago1 tapado" class="Bool (strict)"("Visible"=FALSE) -> ()  [unwired: 2 in, 2 out]
        n1211 = local write "ROJO"(FALSE ("ROJO")) -> ()
        n1212 = local write "AZUL"(FALSE ("AZUL")) -> ()
        n1213 = local write "PESO\nSI"(FALSE ("PESO\nSI")) -> ()
        n1214 = property on="cilindro1 tapado" class="Bool (strict)"("Visible"=FALSE) -> ()  [unwired: 2 in, 2 out]
        n1215 = property on="vastago2 tapado" class="Bool (strict)"("Visible"=FALSE) -> ()  [unwired: 2 in, 2 out]
        n1216 = property on="CILINDRO RECHAZO1" class="Bool (strict)"("Visible"=FALSE) -> ()  [unwired: 2 in, 2 out]
        n1217 = property on="cilindro2 tapado" class="Bool (strict)"("Visible"=FALSE) -> ()  [unwired: 2 in, 2 out]
        n1218 = property on="TAPA NOCOLOR" class="Bool (strict)"("Visible"=FALSE) -> ()  [unwired: 2 in, 2 out]
        n1219 = property on="CILINDRO RECHAZO" class="Bool (strict)"("Visible"=FALSE) -> ()  [unwired: 2 in, 2 out]
        n1220 = property on="vastago3 tapado" class="Bool (strict)"("Visible"=FALSE) -> ()  [unwired: 2 in, 2 out]
        n1221 = property on="cilindro3 tapado" class="Bool (strict)"("Visible"=FALSE) -> ()  [unwired: 2 in, 2 out]
        n1222 = property on="TARRO NOCOLOR" class="Bool (strict)"("Top"=409 ("Position:Top")) -> ()  [unwired: 2 in, 2 out]
        n1223 = property on="vastago4 tapado" class="Bool (strict)"("Visible"=FALSE) -> ()  [unwired: 2 in, 2 out]
        n1224 = property on="vastago3 tapado" class="Bool (strict)"("Top"=206 ("Position:Top")) -> ()  [unwired: 2 in, 2 out]
        n1225 = property on="vastago4 tapado" class="Bool (strict)"("Top"=226 ("Position:Top")) -> ()  [unwired: 2 in, 2 out]
        n1226 = property on="vastago2 tapado" class="Bool (strict)"("Left"=626 ("Position:Left")) -> ()  [unwired: 2 in, 2 out]
        n1227 = property on="CILINDRO RECHAZO" class="Bool (strict)"("Left"=592 ("Position:Left")) -> ()  [unwired: 2 in, 2 out]
        n1228 = property on="CILINDRO RECHAZO1" class="Bool (strict)"("Left"=620 ("Position:Left")) -> ()  [unwired: 2 in, 2 out]
        n1229 = property on="puerta tolva2" class="Bool (strict)"("Left"=450 ("Position:Left")) -> ()  [unwired: 2 in, 2 out]
        n1230 = property on="perta tolva1" class="Bool (strict)"("Left"=450 ("Position:Left")) -> ()  [unwired: 2 in, 2 out]
        n1231 = property on="VASTAGO RECHAZO" class="Bool (strict)"("Left"=614 ("Position:Left")) -> ()  [unwired: 2 in, 2 out]
        n1232 = property on="TAPA TARRO ROJO" class="Bool (strict)"("Top"=14 ("Position:Top")) -> ()  [unwired: 2 in, 2 out]
        n1233 = property on="TAPA TARRO ROJO" class="Bool (strict)"("Left"=916 ("Position:Left")) -> ()  [unwired: 2 in, 2 out]
        n1234 = local write "ANALIZANDO\nCC"(FALSE ("ANALIZANDO\nCC")) -> ()
        n1235 = local write "NO \nCOLOR"(FALSE ("NO \nCOLOR")) -> ()
        n1236 = local write "PESO\nNO"(FALSE ("PESO\nNO")) -> ()
        n1237 = property on="PINZA CERRADA" class="Bool (strict)"("Visible"=FALSE) -> ()  [unwired: 2 in, 2 out]
        n1238 = property on="ESTRUCTURA RECHAZO" class="Bool (strict)"("Visible"=FALSE) -> ()  [unwired: 2 in, 2 out]
        n1239 = property on="PINZA CERRADA" class="Bool (strict)"("Top"=316 ("Position:Top")) -> ()  [unwired: 2 in, 2 out]
        n1240 = property on="TAPA NOPESO" class="Bool (strict)"("Top"=14 ("Position:Top")) -> ()  [unwired: 2 in, 2 out]
        n1241 = property on="TARRO NOPESO" class="Bool (strict)"("Top"=409 ("Position:Top")) -> ()  [unwired: 2 in, 2 out]
        n1242 = property on="VASTAGO RECHAZO" class="Bool (strict)"("Top"=180 ("Position:Top")) -> ()  [unwired: 2 in, 2 out]
        n1243 = property on="PINZA CERRADA" class="Bool (strict)"("Left"=596 ("Position:Left")) -> ()  [unwired: 2 in, 2 out]
        n1244 = property on="TARRO NOPESO" class="Bool (strict)"("Left"=386 ("Position:Left")) -> ()  [unwired: 2 in, 2 out]
        n1245 = property on="TAPA NOPESO" class="Bool (strict)"("Left"=917 ("Position:Left")) -> ()  [unwired: 2 in, 2 out]
        n1246 = local write "M19"(FALSE ("M19")) -> ()
        n1247 = local write "M12"(FALSE ("M12")) -> ()
        n1248 = local write "M13"(FALSE ("M13")) -> ()
        n1249 = local write "M14"(FALSE ("M14")) -> ()
        n1250 = local write "M15"(FALSE ("M15")) -> ()
        n1251 = local write "M16"(FALSE ("M16")) -> ()
        n1252 = local write "M17"(FALSE ("M17")) -> ()
        n1253 = local write "M18"(FALSE ("M18")) -> ()
        n1254 = local write "M10"(FALSE ("M10")) -> ()
        n1255 = local write "M11"(FALSE ("M11")) -> ()
        n1256 = local write "M9"(FALSE ("M9")) -> ()
        n1257 = local write "M6"(FALSE ("M6")) -> ()
        n1258 = local write "M7"(FALSE ("M7")) -> ()
        n1259 = local write "M8"(FALSE ("M8")) -> ()
        n1260 = local write "M3"(FALSE ("M3")) -> ()
        n1261 = local write "M4"(FALSE ("M4")) -> ()
        n1262 = local write "M5"(FALSE ("M5")) -> ()
        n1263 = local write "M2"(FALSE ("M2")) -> ()
        n1264 = local write "M1"(FALSE ("M1")) -> ()
        n1265 = property on="DEPOSITO NOPESO" class="Bool (strict)"("Visible"=FALSE) -> ()  [unwired: 2 in, 2 out]
        n1266 = property on="DEPOSITO NOCOLOR" class="Bool (strict)"("Visible"=FALSE) -> ()  [unwired: 2 in, 2 out]
        n1267 = local write "M27"(FALSE ("M27")) -> ()
        n1268 = local write "M34"(FALSE ("M34")) -> ()
        n1269 = local write "M26"(FALSE ("M26")) -> ()
        n1270 = local write "M30"(FALSE ("M30")) -> ()
        n1271 = local write "M31"(FALSE ("M31")) -> ()
        n1272 = local write "M32"(FALSE ("M32")) -> ()
        n1273 = local write "M33"(FALSE ("M33")) -> ()
        n1274 = local write "M24"(FALSE ("M24")) -> ()
        n1275 = local write "M25"(FALSE ("M25")) -> ()
        n1276 = local write "M28"(FALSE ("M28")) -> ()
        n1277 = local write "M29"(FALSE ("M29")) -> ()
        n1278 = local write "M21"(FALSE ("M21")) -> ()
        n1279 = local write "M23"(FALSE ("M23")) -> ()
        n1280 = local write "M35"(FALSE ("M35")) -> ()
        n1281 = local write "M20"(FALSE ("M20")) -> ()
        n1282 = local write "M22"(FALSE ("M22")) -> ()
        n1283 = local write "M36"(FALSE ("M36")) -> ()
        n1284 = local write "M54"(FALSE ("M54")) -> ()
        n1285 = local write "M43"(FALSE ("M43")) -> ()
        n1286 = local write "M44"(FALSE ("M44")) -> ()
        n1287 = local write "M51"(FALSE ("M51")) -> ()
        n1288 = local write "M52"(FALSE ("M52")) -> ()
        n1289 = local write "M53"(FALSE ("M53")) -> ()
        n1290 = local write "M41"(FALSE ("M41")) -> ()
        n1291 = local write "M42"(FALSE ("M42")) -> ()
        n1292 = local write "M50"(FALSE ("M50")) -> ()
        n1293 = local write "M38"(FALSE ("M38")) -> ()
        n1294 = local write "M39"(FALSE ("M39")) -> ()
        n1295 = local write "M40"(FALSE ("M40")) -> ()
        n1296 = local write "M45"(FALSE ("M45")) -> ()
        n1297 = local write "M49"(FALSE ("M49")) -> ()
        n1298 = local write "M37"(FALSE ("M37")) -> ()
        n1299 = local write "M46"(FALSE ("M46")) -> ()
        n1300 = local write "M48"(FALSE ("M48")) -> ()
        n1301 = local write "M47"(FALSE ("M47")) -> ()
      }
    }
    n1302 = case shown="True" w156 {
      frame False {
      }
      frame True {
        n1303 = property on="PINZA CERRADA" class="Bool (strict)"("Visible"=FALSE) -> ()  [unwired: 2 in, 2 out]
        n1304 = property on="PINZA ABIERTA" class="Bool (strict)"("Visible"=TRUE) -> ()  [unwired: 2 in, 2 out]
        n1305 = local read "FINALIZADOS\nRECHAZADOS"() -> (w636:dbl)
        n1306 = Increment(x=w636) -> (x+1=w635:dbl)
        n1307 = local write "FINALIZADOS\nRECHAZADOS"(w635) -> ()
        n1308 = while {
          stop <- w642 stop-if-true
          n1309 = property on="PINZA ABIERTA" class="Bool (strict)"() -> ("Top"=w656:i32)  [unwired: 2 in, 2 out]
          n1310 = Subtract(x=w656, y=6) -> (x-y=w654:i32)
          n1311 = property on="PINZA ABIERTA" class="Bool (strict)"("Top"=w654) -> ()  [unwired: 2 in, 2 out]
          n1312 = property on="VASTAGO RECHAZO" class="Bool (strict)"() -> ("Top"=w653:i32)  [unwired: 2 in, 2 out]
          n1313 = Subtract(x=w653, y=6) -> (x-y=w651:i32)
          n1314 = property on="VASTAGO RECHAZO" class="Bool (strict)"("Top"=w651) -> ()  [unwired: 2 in, 2 out]
          n1315 = property on="PINZA CERRADA" class="Bool (strict)"() -> ("Top"=w650:i32)  [unwired: 2 in, 2 out]
          n1316 = Subtract(x=w650, y=6) -> (x-y=w648:i32)
          n1317 = property on="PINZA CERRADA" class="Bool (strict)"("Top"=w648) -> ()  [unwired: 2 in, 2 out]
          n1318 = Wait (ms)(milliseconds to wait=u32 0) -> ()  [unwired: 1 out]
          n1319 = local read "RESET"() -> (w643:bool)
          n1320 = property on="PINZA CERRADA" class="Bool (strict)"() -> ("Top"=w646:i32)  [unwired: 2 in, 2 out]
          n1321 = Less?(x=w646, y=317) -> (x < y?=w644:bool)
          n1322 = Or(x=w644, y=w643) -> (x .or. y?=w642:bool)
        }
        n1323 = local write "NO \nCOLOR"(FALSE ("NO \nCOLOR")) -> ()
        n1324 = local write "M42"(FALSE ("M42")) -> ()
        n1325 = local write "M43"(TRUE ("M43")) -> ()
      }
    }
    n1326 = case shown="True" w99 {
      frame False {
      }
      frame True {
        n1327 = property on="PINZA ABIERTA" class="Bool (strict)"("Visible"=TRUE) -> ()  [unwired: 2 in, 2 out]
        n1328 = property on="PINZA CERRADA" class="Bool (strict)"("Visible"=FALSE) -> ()  [unwired: 2 in, 2 out]
        n1329 = local read "FINALIZADOS\nRECHAZADOS"() -> (w414:dbl)
        n1330 = Increment(x=w414) -> (x+1=w413:dbl)
        n1331 = local write "FINALIZADOS\nRECHAZADOS"(w413) -> ()
        n1332 = while {
          stop <- w417 stop-if-true
          n1333 = property on="PINZA ABIERTA" class="Bool (strict)"() -> ("Top"=w431:i32)  [unwired: 2 in, 2 out]
          n1334 = Subtract(x=w431, y=6) -> (x-y=w429:i32)
          n1335 = property on="PINZA ABIERTA" class="Bool (strict)"("Top"=w429) -> ()  [unwired: 2 in, 2 out]
          n1336 = property on="VASTAGO RECHAZO" class="Bool (strict)"() -> ("Top"=w428:i32)  [unwired: 2 in, 2 out]
          n1337 = Subtract(x=w428, y=6) -> (x-y=w426:i32)
          n1338 = property on="VASTAGO RECHAZO" class="Bool (strict)"("Top"=w426) -> ()  [unwired: 2 in, 2 out]
          n1339 = property on="PINZA CERRADA" class="Bool (strict)"() -> ("Top"=w425:i32)  [unwired: 2 in, 2 out]
          n1340 = Subtract(x=w425, y=6) -> (x-y=w423:i32)
          n1341 = property on="PINZA CERRADA" class="Bool (strict)"("Top"=w423) -> ()  [unwired: 2 in, 2 out]
          n1342 = Wait (ms)(milliseconds to wait=u32 0) -> ()  [unwired: 1 out]
          n1343 = local read "RESET"() -> (w418:bool)
          n1344 = property on="PINZA CERRADA" class="Bool (strict)"() -> ("Top"=w421:i32)  [unwired: 2 in, 2 out]
          n1345 = Less?(x=w421, y=317) -> (x < y?=w419:bool)
          n1346 = Or(x=w419, y=w418) -> (x .or. y?=w417:bool)
        }
        n1347 = local write "PESO\nNO"(FALSE ("PESO\nNO")) -> ()
        n1348 = local write "M53"(TRUE ("M53")) -> ()
        n1349 = local write "M52"(FALSE ("M52")) -> ()
      }
    }
    n1350 = case shown="True" w94 {
      frame False {
      }
      frame True {
        n1351 = while {
          stop <- w386 stop-if-true
          n1352 = property on="PINZA ABIERTA" class="Bool (strict)"() -> ("Left"=w409:i32)  [unwired: 2 in, 2 out]
          n1353 = Add(x=w409, y=9) -> (x+y=w407:i32)
          n1354 = property on="PINZA ABIERTA" class="Bool (strict)"("Left"=w407) -> ()  [unwired: 2 in, 2 out]
          n1355 = property on="VASTAGO RECHAZO" class="Bool (strict)"() -> ("Left"=w406:i32)  [unwired: 2 in, 2 out]
          n1356 = Add(x=w406, y=9) -> (x+y=w404:i32)
          n1357 = property on="VASTAGO RECHAZO" class="Bool (strict)"("Left"=w404) -> ()  [unwired: 2 in, 2 out]
          n1358 = property on="CILINDRO RECHAZO" class="Bool (strict)"() -> ("Left"=w403:i32)  [unwired: 2 in, 2 out]
          n1359 = Add(x=w403, y=9) -> (x+y=w401:i32)
          n1360 = property on="CILINDRO RECHAZO" class="Bool (strict)"("Left"=w401) -> ()  [unwired: 2 in, 2 out]
          n1361 = property on="CILINDRO RECHAZO1" class="Bool (strict)"() -> ("Left"=w400:i32)  [unwired: 2 in, 2 out]
          n1362 = Add(x=w400, y=9) -> (x+y=w398:i32)
          n1363 = property on="CILINDRO RECHAZO1" class="Bool (strict)"("Left"=w398) -> ()  [unwired: 2 in, 2 out]
          n1364 = property on="PINZA CERRADA" class="Bool (strict)"() -> ("Left"=w397:i32)  [unwired: 2 in, 2 out]
          n1365 = Add(x=w397, y=9) -> (x+y=w395:i32)
          n1366 = property on="PINZA CERRADA" class="Bool (strict)"("Left"=w395) -> ()  [unwired: 2 in, 2 out]
          n1367 = property on="ACTUADOR RECHAZO" class="Bool (strict)"() -> ("Top"=w394:i32)  [unwired: 2 in, 2 out]
          n1368 = Add(x=w394, y=9) -> (x+y=w392:i32)
          n1369 = property on="ACTUADOR RECHAZO" class="Bool (strict)"("Top"=w392) -> ()  [unwired: 2 in, 2 out]
          n1370 = Wait (ms)(milliseconds to wait=u32 0) -> ()  [unwired: 1 out]
          n1371 = local read "RESET"() -> (w387:bool)
          n1372 = property on="ACTUADOR RECHAZO" class="Bool (strict)"() -> ("Top"=w390:i32)  [unwired: 2 in, 2 out]
          n1373 = Greater?(x=w390, y=219) -> (0:w388:bool)
          n1374 = Or(x=w388, y=w387) -> (x .or. y?=w386:bool)
        }
        n1375 = local write "M53"(FALSE ("M53")) -> ()
        n1376 = local write "M54"(TRUE ("M54")) -> ()
      }
    }
    n1377 = property on="BNO COLOR" class="Bool (strict)"("Visible"=FALSE) -> ()  [unwired: 2 in, 2 out]
    n1378 = property on="BPESO SI" class="Bool (strict)"("Visible"=FALSE) -> ()  [unwired: 2 in, 2 out]
    n1379 = local write "BAZUL"(w65) -> ()
    n1380 = local write "BROJO"(w64) -> ()
    n1381 = local write "BNO COLOR"(w68) -> ()
    n1382 = local write "BPESO NO"(w67) -> ()
    n1383 = local write "BPESO SI"(w66) -> ()
    n1384 = case shown="True" w332 {
      frame False {
      }
      frame True {
        n1385 = property on="estructura tapado" class="Bool (strict)"("Visible"=TRUE) -> ()  [unwired: 2 in, 2 out]
        n1386 = property on="tapa neutrop" class="Bool (strict)"("Visible"=TRUE) -> ()  [unwired: 2 in, 2 out]
        n1387 = property on="vastago1 tapado" class="Bool (strict)"("Visible"=TRUE) -> ()  [unwired: 2 in, 2 out]
        n1388 = property on="cilindro1 tapado" class="Bool (strict)"("Visible"=TRUE) -> ()  [unwired: 2 in, 2 out]
        n1389 = property on="vastago2 tapado" class="Bool (strict)"("Visible"=TRUE) -> ()  [unwired: 2 in, 2 out]
        n1390 = property on="cilindro2 tapado" class="Bool (strict)"("Visible"=TRUE) -> ()  [unwired: 2 in, 2 out]
        n1391 = property on="vastago3 tapado" class="Bool (strict)"("Visible"=TRUE) -> ()  [unwired: 2 in, 2 out]
        n1392 = property on="cilindro3 tapado" class="Bool (strict)"("Visible"=TRUE) -> ()  [unwired: 2 in, 2 out]
        n1393 = property on="vastago4 tapado" class="Bool (strict)"("Visible"=TRUE) -> ()  [unwired: 2 in, 2 out]
        n1394 = while {
          stop <- w1218 stop-if-true
          n1395 = property on="CILINDRO NUEVO" class="Bool (strict)"() -> ("Left"=w1241:i32)  [unwired: 2 in, 2 out]
          n1396 = Add(x=w1241, y=1) -> (x+y=w1219:i32)
          n1397 = property on="CILINDRO NUEVO" class="Bool (strict)"("Left"=w1219) -> ()  [unwired: 2 in, 2 out]
          n1398 = property on="BASTAGO TAPAS" class="Bool (strict)"() -> ("Left"=w1239:i32)  [unwired: 2 in, 2 out]
          n1399 = Subtract(x=w1239, y=3) -> (x-y=w1236:i32)
          n1400 = property on="BASTAGO TAPAS" class="Bool (strict)"("Left"=w1236) -> ()  [unwired: 2 in, 2 out]
          n1401 = property on="TAPA NEUTRO" class="Bool (strict)"() -> ("Left"=w1234:i32)  [unwired: 2 in, 2 out]
          n1402 = Subtract(x=w1234, y=3) -> (x-y=w1232:i32)
          n1403 = property on="TAPA NEUTRO" class="Bool (strict)"("Left"=w1232) -> ()  [unwired: 2 in, 2 out]
          n1404 = property on="vastago1 tapado" class="Bool (strict)"() -> ("Left"=w1229:i32)  [unwired: 2 in, 2 out]
          n1405 = Add(x=w1229, y=3) -> (x+y=w1227:i32)
          n1406 = property on="vastago1 tapado" class="Bool (strict)"("Left"=w1227) -> ()  [unwired: 2 in, 2 out]
          n1407 = property on="tapa neutrop" class="Bool (strict)"() -> ("Left"=w1226:i32)  [unwired: 2 in, 2 out]
          n1408 = Add(x=w1226, y=3) -> (x+y=w1224:i32)
          n1409 = property on="tapa neutrop" class="Bool (strict)"("Left"=w1224) -> ()  [unwired: 2 in, 2 out]
          n1410 = property on="vastago2 tapado" class="Bool (strict)"() -> ("Left"=w1223:i32)  [unwired: 2 in, 2 out]
          n1411 = Subtract(x=w1223, y=1) -> (x-y=w1221:i32)
          n1412 = property on="vastago2 tapado" class="Bool (strict)"("Left"=w1221) -> ()  [unwired: 2 in, 2 out]
          n1413 = Wait (ms)(milliseconds to wait=u32 0) -> ()  [unwired: 1 out]
          n1414 = local read "RESET"() -> (w1230:bool)
          n1415 = property on="BASTAGO TAPAS" class="Bool (strict)"() -> ("Left"=w1235:i32)  [unwired: 2 in, 2 out]
          n1416 = Less?(x=w1235, y=911) -> (x < y?=w1231:bool)
          n1417 = Or(x=w1231, y=w1230) -> (x .or. y?=w1218:bool)
        }
        n1418 = local write "M9"(FALSE ("M9")) -> ()
        n1419 = local write "M10"(TRUE ("M10")) -> ()
      }
    }
    n1420 = case shown="True" w181 {
      frame False {
      }
      frame True {
        n1421 = property on="CILINDRO RECHAZO1" class="Bool (strict)"("Visible"=TRUE) -> ()  [unwired: 2 in, 2 out]
        n1422 = property on="ESTRUCTURA RECHAZO" class="Bool (strict)"("Visible"=TRUE) -> ()  [unwired: 2 in, 2 out]
        n1423 = property on="CILINDRO RECHAZO" class="Bool (strict)"("Visible"=TRUE) -> ()  [unwired: 2 in, 2 out]
        n1424 = property on="TARRO NOCOLOR" class="Bool (strict)"("Visible"=TRUE) -> ()  [unwired: 2 in, 2 out]
        n1425 = property on="PINZA ABIERTA" class="Bool (strict)"("Visible"=TRUE) -> ()  [unwired: 2 in, 2 out]
        n1426 = property on="VASTAGO RECHAZO" class="Bool (strict)"("Visible"=TRUE) -> ()  [unwired: 2 in, 2 out]
        n1427 = property on="DEPOSITO NOCOLOR" class="Bool (strict)"("Visible"=TRUE) -> ()  [unwired: 2 in, 2 out]
        n1428 = property on="DEPOSITO NOPESO" class="Bool (strict)"("Visible"=TRUE) -> ()  [unwired: 2 in, 2 out]
        n1429 = while {
          stop <- w757 stop-if-true
          n1430 = property on="CILINDRO RECHAZO1" class="Bool (strict)"() -> ("Left"=w780:i32)  [unwired: 2 in, 2 out]
          n1431 = Subtract(x=w780, y=9) -> (x-y=w778:i32)
          n1432 = property on="CILINDRO RECHAZO1" class="Bool (strict)"("Left"=w778) -> ()  [unwired: 2 in, 2 out]
          n1433 = property on="PINZA CERRADA" class="Bool (strict)"() -> ("Left"=w777:i32)  [unwired: 2 in, 2 out]
          n1434 = Subtract(x=w777, y=9) -> (x-y=w775:i32)
          n1435 = property on="PINZA CERRADA" class="Bool (strict)"("Left"=w775) -> ()  [unwired: 2 in, 2 out]
          n1436 = property on="CILINDRO RECHAZO" class="Bool (strict)"() -> ("Left"=w774:i32)  [unwired: 2 in, 2 out]
          n1437 = Subtract(x=w774, y=9) -> (x-y=w772:i32)
          n1438 = property on="CILINDRO RECHAZO" class="Bool (strict)"("Left"=w772) -> ()  [unwired: 2 in, 2 out]
          n1439 = property on="VASTAGO RECHAZO" class="Bool (strict)"() -> ("Left"=w771:i32)  [unwired: 2 in, 2 out]
          n1440 = Subtract(x=w771, y=9) -> (x-y=w769:i32)
          n1441 = property on="VASTAGO RECHAZO" class="Bool (strict)"("Left"=w769) -> ()  [unwired: 2 in, 2 out]
          n1442 = property on="PINZA ABIERTA" class="Bool (strict)"() -> ("Left"=w768:i32)  [unwired: 2 in, 2 out]
          n1443 = Subtract(x=w768, y=9) -> (x-y=w766:i32)
          n1444 = property on="PINZA ABIERTA" class="Bool (strict)"("Left"=w766) -> ()  [unwired: 2 in, 2 out]
          n1445 = property on="ACTUADOR RECHAZO" class="Bool (strict)"() -> ("Top"=w765:i32)  [unwired: 2 in, 2 out]
          n1446 = Subtract(x=w765, y=9) -> (x-y=w763:i32)
          n1447 = property on="ACTUADOR RECHAZO" class="Bool (strict)"("Top"=w763) -> ()  [unwired: 2 in, 2 out]
          n1448 = Wait (ms)(milliseconds to wait=u32 0) -> ()  [unwired: 1 out]
          n1449 = local read "RESET"() -> (w758:bool)
          n1450 = property on="ACTUADOR RECHAZO" class="Bool (strict)"() -> ("Top"=w761:i32)  [unwired: 2 in, 2 out]
          n1451 = Less?(x=w761, y=6) -> (x < y?=w759:bool)
          n1452 = Or(x=w759, y=w758) -> (x .or. y?=w757:bool)
        }
        n1453 = local write "M37"(FALSE ("M37")) -> ()
        n1454 = local write "M38"(TRUE ("M38")) -> ()
      }
    }
    n1455 = case shown="True" w166 {
      frame False {
      }
      frame True {
        n1456 = while {
          stop <- w679 stop-if-true
          n1457 = property on="PINZA ABIERTA" class="Bool (strict)"() -> ("Left"=w708:i32)  [unwired: 2 in, 2 out]
          n1458 = Add(x=w708, y=12) -> (x+y=w706:i32)
          n1459 = property on="PINZA ABIERTA" class="Bool (strict)"("Left"=w706) -> ()  [unwired: 2 in, 2 out]
          n1460 = property on="VASTAGO RECHAZO" class="Bool (strict)"() -> ("Left"=w705:i32)  [unwired: 2 in, 2 out]
          n1461 = Add(x=w705, y=12) -> (x+y=w703:i32)
          n1462 = property on="VASTAGO RECHAZO" class="Bool (strict)"("Left"=w703) -> ()  [unwired: 2 in, 2 out]
          n1463 = property on="TARRO NOCOLOR" class="Bool (strict)"() -> ("Left"=w702:i32)  [unwired: 2 in, 2 out]
          n1464 = Add(x=w702, y=12) -> (x+y=w700:i32)
          n1465 = property on="TARRO NOCOLOR" class="Bool (strict)"("Left"=w700) -> ()  [unwired: 2 in, 2 out]
          n1466 = property on="TAPA NOCOLOR" class="Bool (strict)"() -> ("Top"=w699:i32)  [unwired: 2 in, 2 out]
          n1467 = Add(x=w699, y=12) -> (x+y=w697:i32)
          n1468 = property on="TAPA NOCOLOR" class="Bool (strict)"("Top"=w697) -> ()  [unwired: 2 in, 2 out]
          n1469 = property on="CILINDRO RECHAZO" class="Bool (strict)"() -> ("Left"=w696:i32)  [unwired: 2 in, 2 out]
          n1470 = Add(x=w696, y=12) -> (x+y=w694:i32)
          n1471 = property on="CILINDRO RECHAZO" class="Bool (strict)"("Left"=w694) -> ()  [unwired: 2 in, 2 out]
          n1472 = property on="PINZA CERRADA" class="Bool (strict)"() -> ("Left"=w693:i32)  [unwired: 2 in, 2 out]
          n1473 = Add(x=w693, y=12) -> (x+y=w691:i32)
          n1474 = property on="PINZA CERRADA" class="Bool (strict)"("Left"=w691) -> ()  [unwired: 2 in, 2 out]
          n1475 = property on="CILINDRO RECHAZO1" class="Bool (strict)"() -> ("Left"=w690:i32)  [unwired: 2 in, 2 out]
          n1476 = Add(x=w690, y=12) -> (x+y=w688:i32)
          n1477 = property on="CILINDRO RECHAZO1" class="Bool (strict)"("Left"=w688) -> ()  [unwired: 2 in, 2 out]
          n1478 = property on="ACTUADOR RECHAZO" class="Bool (strict)"() -> ("Top"=w687:i32)  [unwired: 2 in, 2 out]
          n1479 = Add(x=w687, y=12) -> (x+y=w685:i32)
          n1480 = property on="ACTUADOR RECHAZO" class="Bool (strict)"("Top"=w685) -> ()  [unwired: 2 in, 2 out]
          n1481 = Wait (ms)(milliseconds to wait=u32 0) -> ()  [unwired: 1 out]
          n1482 = local read "RESET"() -> (w680:bool)
          n1483 = property on="ACTUADOR RECHAZO" class="Bool (strict)"() -> ("Top"=w683:i32)  [unwired: 2 in, 2 out]
          n1484 = Greater?(x=w683, y=219) -> (0:w681:bool)
          n1485 = Or(x=w681, y=w680) -> (x .or. y?=w679:bool)
        }
        n1486 = local write "M40"(FALSE ("M40")) -> ()
        n1487 = local write "M41"(TRUE ("M41")) -> ()
      }
    }
    n1488 = case shown="True" w124 {
      frame False {
      }
      frame True {
        n1489 = property on="CILINDRO RECHAZO1" class="Bool (strict)"("Visible"=TRUE) -> ()  [unwired: 2 in, 2 out]
        n1490 = property on="ESTRUCTURA RECHAZO" class="Bool (strict)"("Visible"=TRUE) -> ()  [unwired: 2 in, 2 out]
        n1491 = property on="CILINDRO RECHAZO" class="Bool (strict)"("Visible"=TRUE) -> ()  [unwired: 2 in, 2 out]
        n1492 = property on="TARRO NOPESO" class="Bool (strict)"("Visible"=TRUE) -> ()  [unwired: 2 in, 2 out]
        n1493 = property on="PINZA ABIERTA" class="Bool (strict)"("Visible"=TRUE) -> ()  [unwired: 2 in, 2 out]
        n1494 = property on="VASTAGO RECHAZO" class="Bool (strict)"("Visible"=TRUE) -> ()  [unwired: 2 in, 2 out]
        n1495 = property on="DEPOSITO NOCOLOR" class="Bool (strict)"("Visible"=TRUE) -> ()  [unwired: 2 in, 2 out]
        n1496 = property on="DEPOSITO NOPESO" class="Bool (strict)"("Visible"=TRUE) -> ()  [unwired: 2 in, 2 out]
        n1497 = while {
          stop <- w536 stop-if-true
          n1498 = property on="CILINDRO RECHAZO1" class="Bool (strict)"() -> ("Left"=w556:i32)  [unwired: 2 in, 2 out]
          n1499 = Subtract(x=w556, y=9) -> (x-y=w554:i32)
          n1500 = property on="CILINDRO RECHAZO1" class="Bool (strict)"("Left"=w554) -> ()  [unwired: 2 in, 2 out]
          n1501 = property on="PINZA CERRADA" class="Bool (strict)"() -> ("Left"=w553:i32)  [unwired: 2 in, 2 out]
          n1502 = Subtract(x=w553, y=9) -> (x-y=w551:i32)
          n1503 = property on="PINZA CERRADA" class="Bool (strict)"("Left"=w551) -> ()  [unwired: 2 in, 2 out]
          n1504 = property on="CILINDRO RECHAZO" class="Bool (strict)"() -> ("Left"=w550:i32)  [unwired: 2 in, 2 out]
          n1505 = Subtract(x=w550, y=9) -> (x-y=w548:i32)
          n1506 = property on="CILINDRO RECHAZO" class="Bool (strict)"("Left"=w548) -> ()  [unwired: 2 in, 2 out]
          n1507 = property on="VASTAGO RECHAZO" class="Bool (strict)"() -> ("Left"=w547:i32)  [unwired: 2 in, 2 out]
          n1508 = Subtract(x=w547, y=9) -> (x-y=w545:i32)
          n1509 = property on="VASTAGO RECHAZO" class="Bool (strict)"("Left"=w545) -> ()  [unwired: 2 in, 2 out]
          n1510 = property on="PINZA ABIERTA" class="Bool (strict)"() -> ("Left"=w544:i32)  [unwired: 2 in, 2 out]
          n1511 = Subtract(x=w544, y=9) -> (x-y=w542:i32)
          n1512 = property on="PINZA ABIERTA" class="Bool (strict)"("Left"=w542) -> ()  [unwired: 2 in, 2 out]
          n1513 = property on="ACTUADOR RECHAZO" class="Bool (strict)"() -> ("Top"=w535:i32)  [unwired: 2 in, 2 out]
          n1514 = Subtract(x=w535, y=9) -> (x-y=w534:i32)
          n1515 = property on="ACTUADOR RECHAZO" class="Bool (strict)"("Top"=w534) -> ()  [unwired: 2 in, 2 out]
          n1516 = Wait (ms)(milliseconds to wait=u32 0) -> ()  [unwired: 1 out]
          n1517 = local read "RESET"() -> (w537:bool)
          n1518 = property on="ACTUADOR RECHAZO" class="Bool (strict)"() -> ("Top"=w533:i32)  [unwired: 2 in, 2 out]
          n1519 = Less?(x=w533, y=6) -> (x < y?=w538:bool)
          n1520 = Or(x=w538, y=w537) -> (x .or. y?=w536:bool)
        }
        n1521 = local write "M47"(FALSE ("M47")) -> ()
        n1522 = local write "M48"(TRUE ("M48")) -> ()
      }
    }
    n1523 = case shown="True" w109 {
      frame False {
      }
      frame True {
        n1524 = while {
          stop <- w456 stop-if-true
          n1525 = property on="PINZA ABIERTA" class="Bool (strict)"() -> ("Left"=w483:i32)  [unwired: 2 in, 2 out]
          n1526 = Add(x=w483, y=9) -> (x+y=w481:i32)
          n1527 = property on="PINZA ABIERTA" class="Bool (strict)"("Left"=w481) -> ()  [unwired: 2 in, 2 out]
          n1528 = property on="VASTAGO RECHAZO" class="Bool (strict)"() -> ("Left"=w480:i32)  [unwired: 2 in, 2 out]
          n1529 = Add(x=w480, y=9) -> (x+y=w478:i32)
          n1530 = property on="VASTAGO RECHAZO" class="Bool (strict)"("Left"=w478) -> ()  [unwired: 2 in, 2 out]
          n1531 = property on="TARRO NOPESO" class="Bool (strict)"() -> ("Left"=w477:i32)  [unwired: 2 in, 2 out]
          n1532 = Add(x=w477, y=9) -> (x+y=w475:i32)
          n1533 = property on="TARRO NOPESO" class="Bool (strict)"("Left"=w475) -> ()  [unwired: 2 in, 2 out]
          n1534 = property on="TAPA NOPESO" class="Bool (strict)"() -> ("Top"=w455:i32)  [unwired: 2 in, 2 out]
          n1535 = Add(x=w455, y=9) -> (x+y=w454:i32)
          n1536 = property on="TAPA NOPESO" class="Bool (strict)"("Top"=w454) -> ()  [unwired: 2 in, 2 out]
          n1537 = property on="CILINDRO RECHAZO" class="Bool (strict)"() -> ("Left"=w473:i32)  [unwired: 2 in, 2 out]
          n1538 = Add(x=w473, y=9) -> (x+y=w471:i32)
          n1539 = property on="CILINDRO RECHAZO" class="Bool (strict)"("Left"=w471) -> ()  [unwired: 2 in, 2 out]
          n1540 = property on="PINZA CERRADA" class="Bool (strict)"() -> ("Left"=w470:i32)  [unwired: 2 in, 2 out]
          n1541 = Add(x=w470, y=9) -> (x+y=w468:i32)
          n1542 = property on="PINZA CERRADA" class="Bool (strict)"("Left"=w468) -> ()  [unwired: 2 in, 2 out]
          n1543 = property on="CILINDRO RECHAZO1" class="Bool (strict)"() -> ("Left"=w467:i32)  [unwired: 2 in, 2 out]
          n1544 = Add(x=w467, y=9) -> (x+y=w465:i32)
          n1545 = property on="CILINDRO RECHAZO1" class="Bool (strict)"("Left"=w465) -> ()  [unwired: 2 in, 2 out]
          n1546 = property on="ACTUADOR RECHAZO" class="Bool (strict)"() -> ("Top"=w464:i32)  [unwired: 2 in, 2 out]
          n1547 = Add(x=w464, y=9) -> (x+y=w462:i32)
          n1548 = property on="ACTUADOR RECHAZO" class="Bool (strict)"("Top"=w462) -> ()  [unwired: 2 in, 2 out]
          n1549 = Wait (ms)(milliseconds to wait=u32 0) -> ()  [unwired: 1 out]
          n1550 = local read "RESET"() -> (w457:bool)
          n1551 = property on="ACTUADOR RECHAZO" class="Bool (strict)"() -> ("Top"=w460:i32)  [unwired: 2 in, 2 out]
          n1552 = Greater?(x=w460, y=100) -> (0:w458:bool)
          n1553 = Or(x=w458, y=w457) -> (x .or. y?=w456:bool)
        }
        n1554 = local write "M50"(FALSE ("M50")) -> ()
        n1555 = local write "M51"(TRUE ("M51")) -> ()
      }
    }
    n1556 = local read "INICIO"() -> (w63:bool)
    n1557 = local read "RESET"() -> (w69:bool)
    n1558 = property on="BPESO NO" class="Bool (strict)"("Visible"=FALSE) -> ()  [unwired: 2 in, 2 out]
    n1559 = Build Array(w63, w69) -> (w70:bool[])
    n1560 = call "DAQ Assistant2"("data"=w70) -> ()  [unwired: 17 in, 2 out]
    n1561 = local read "REINICIAR\nCONTEO"() -> (w373:bool)
    n1562 = case shown="True" w373 {
      frame False {
      }
      frame True {
        n1563 = local read "FINALIZADOS\nAZULES"() -> (w1555:dbl)
        n1564 = local read "FINALIZADOS\nROJOS"() -> (w1557:dbl)
        n1565 = local read "FINALIZADOS\nRECHAZADOS"() -> (w1559:dbl)
        n1566 = Multiply(x=w1555, y=0.0) -> (x*y=w1553:dbl)
        n1567 = Multiply(x=w1557, y=0.0) -> (x*y=w1552:dbl)
        n1568 = Multiply(x=w1559, y=0.0) -> (x*y=w1551:dbl)
        n1569 = local write "FINALIZADOS\nAZULES"(w1553) -> ()
        n1570 = local write "FINALIZADOS\nROJOS"(w1552) -> ()
        n1571 = local write "FINALIZADOS\nRECHAZADOS"(w1551) -> ()
      }
    }
  }
